vi "ScriptedStateMachine.vi"(7 "ScriptSectionName":string="Script", 8 "ErrorArray":errorcluster[](array[cluster]), 10 "script":string[](array[string]), 11 "Test.lvclass":refnum<class "Test.lvclass">) -> (0 "ErrorArray":errorcluster[](array[cluster]), 2 "Data":variant, 3 "Test.lvclass":refnum<class "Test.lvclass">)   [LabVIEW 2018, in "Test.lvclass"]
doc: "This VI sends commands to each module."
uses:
  Test.lvclass
  Test.lvclass/Test.ctl
  Typedef/BdcstInfo.ctl
  Sync/SyncPlugins/SyncPluginBase/Typedefs/clEnaTrigTmstmp.ctl
  Sync/SyncPlugins/SyncPluginBase/Typedefs/clGetTrigTmstmp.ctl
  Scope/ScopePlugins/ScopePluginBaseClass/Typedefs/Sync.ctl
  Accessors/Read ErrorSeverity.vi
  Accessors/Write ErrorSeverity.vi
  Accessors/Read ModuleIDs.vi
  Accessors/Read PluginPathArray.vi
  Accessors/Read PluginIndex.vi
  Accessors/Read LoopScript.vi
  <extravilib>/ChannelInstances/Tag-bool/Read With Abort.vi
  <extravilib>/ChannelInstances/Tag-bool/Write With Abort.vi
  <extravilib>/ChannelInstances/Tag-bool/Instantiate.vi
  <extravilib>/ChannelInstances/Tag-bool/EndpointRead.vi
  <vilib>/Utility/error.llb/Error Cluster From Error Code.vi
  <extravilib>/ChannelInstances/Tag-bool/Endpoint.vi
  <vilib>/ErrorRing/Error Ring.xnode
  <userlib>/NIST/NISTErrorLib/NISTErrorLib.lvlib
  Sync/SyncPlugins/SyncPluginBase/SyncPluginBase.lvclass
  Digitizer/DigitizerPlugins/DigitizerBaseClass/DigitizerBase.lvclass
  Sync/SyncModule/SyncModule.lvlib
  FGen/FgenModule/FgenModule.lvlib
  Digitizer/DigitizerModule/DigitizerModule.lvlib
  FGen/FgenPlugins/FgenPluginBaseClass/FgenPluginsBase.lvclass
  Analysis/AnalysisPlugins/AnalysisPluginBaseClass/AnalysisPluginsBase.lvclass
  Analysis/AnalysisModule/AnalysisModule.lvlib
  Sensor/SensorModule/SensorModule.lvlib
  Scope/ScopeModule/ScopeModule.lvlib
  Scope/ScopePlugins/ScopePluginBaseClass/ScopePluginsBase.lvclass
  AcPwr/AcPwrModule/AcPwrModule.lvlib
  <extravilib>/ChannelInstances/Tag-bool.lvlib
panel:
  out "ErrorSeverity":string
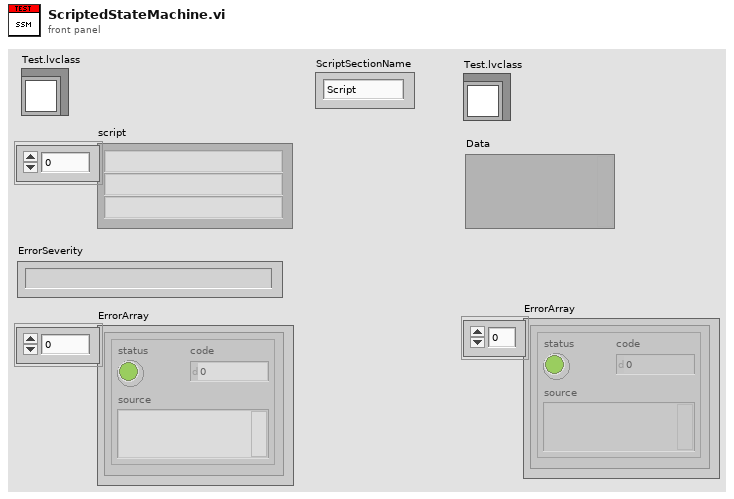
[diagram p1: front panel]
types:
  T1 = typedef "Test.lvclass/BdcstInfo.ctl" = cluster{"ModuleID":i32, "ModuleType":string, "UserEvtRef":variant, "ScriptCmd":string, "Timeout":i32}
  T2 = typedef "SyncPlugins.lvlib/SyncPluginBase.lvclass/clEnaTrigTmstmp.ctl" = cluster{"TriggerName":string, "Enable":bool}
  T3 = typedef "SyncPlugins.lvlib/SyncPluginBase.lvclass/clGetTrigTmstmp.ctl" = cluster{"TriggerName":string, "Timeout (s)":dbl}
  T4 = typedef "ScopePlugins.lvlib/ScopePluginsBase.lvclass/Sync.ctl" = cluster{"Handle":string, "SrcTerm":string, "DestTerm":string}
  T5 = typedef "Test.lvclass/FGenEventReg.ctl" = refnum<event-registration>
  T6 = typedef "Test.lvclass/ScopeEventReg.ctl" = refnum<event-registration>
  T7 = typedef "Test.lvclass/DigitizerEventReg.ctl" = refnum<event-registration>
  T8 = typedef "Test.lvclass/AcPwrEventReg.ctl" = refnum<event-registration>
  T9 = typedef "Tag-bool.lvlib/))Channel.ctl" = refnum<queue>
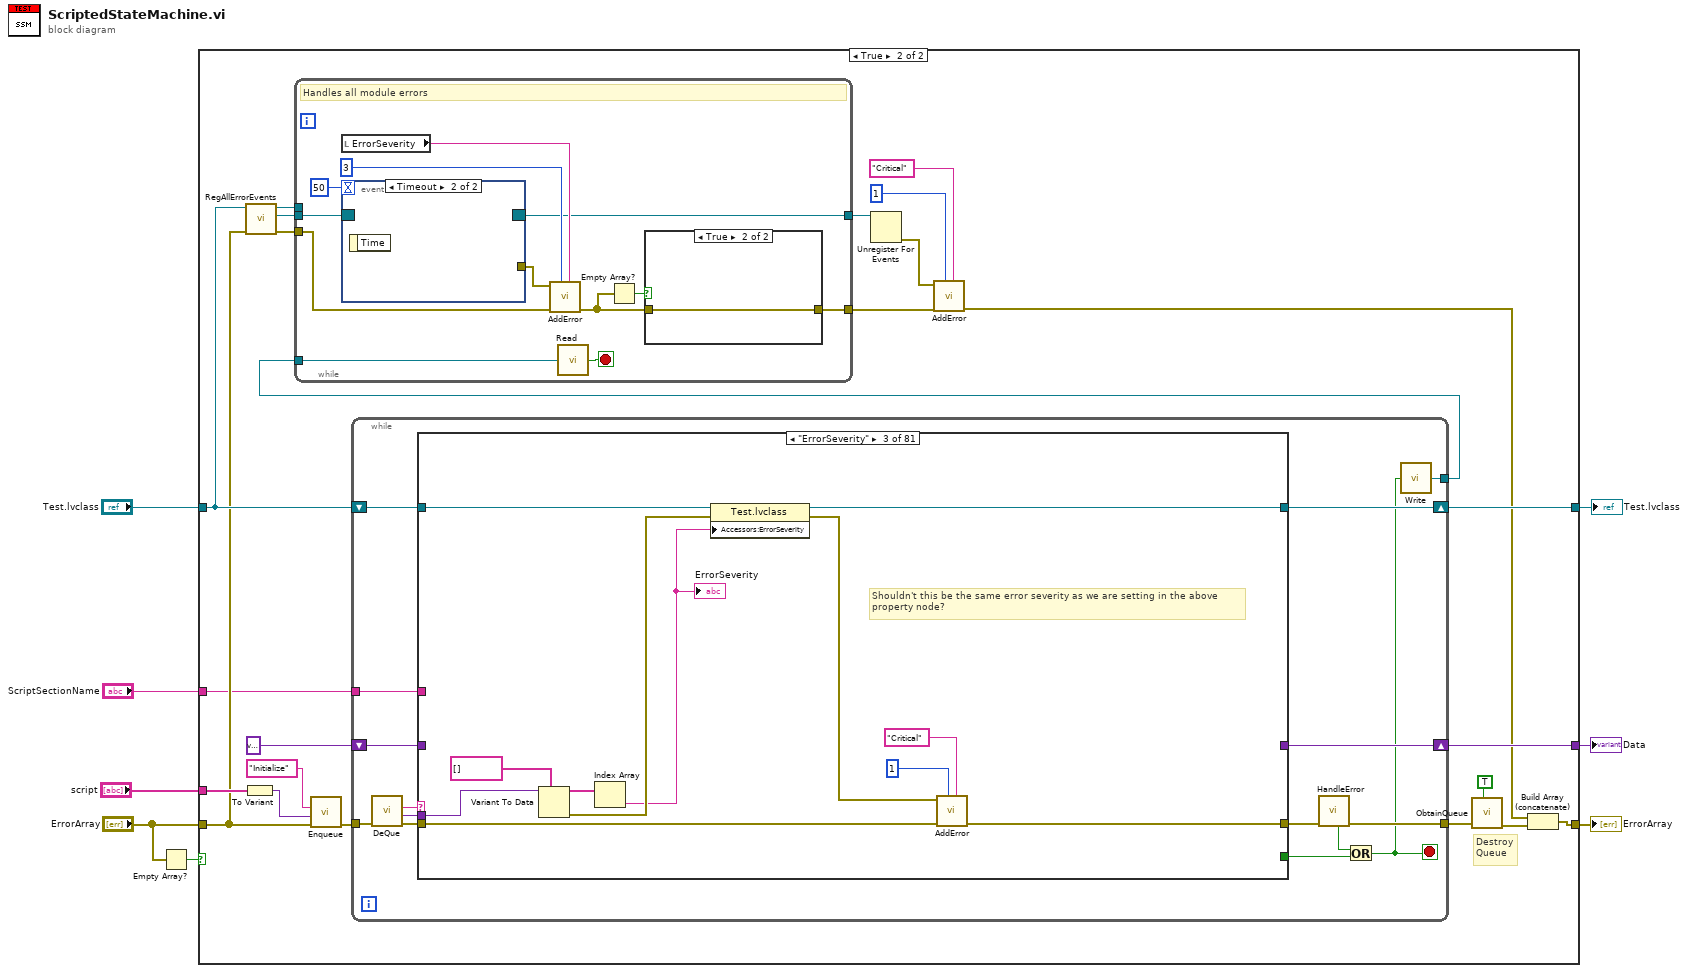
[diagram p0: block diagram]
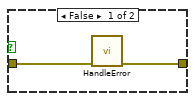
[diagram p3: hidden frame]
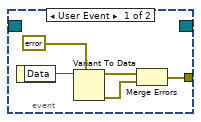
[diagram p4: hidden frame]
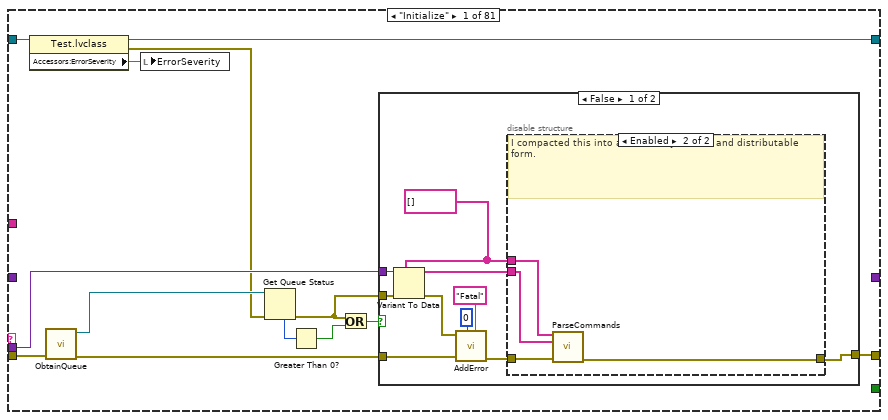
[diagram p5: hidden frame]
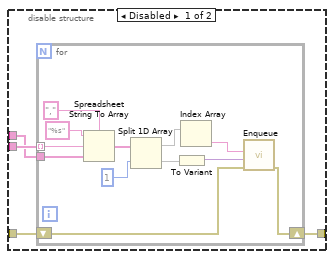
[diagram p6: hidden frame]
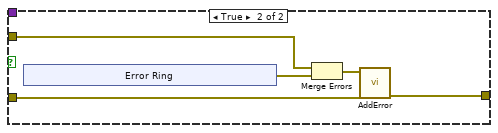
[diagram p7: hidden frame]
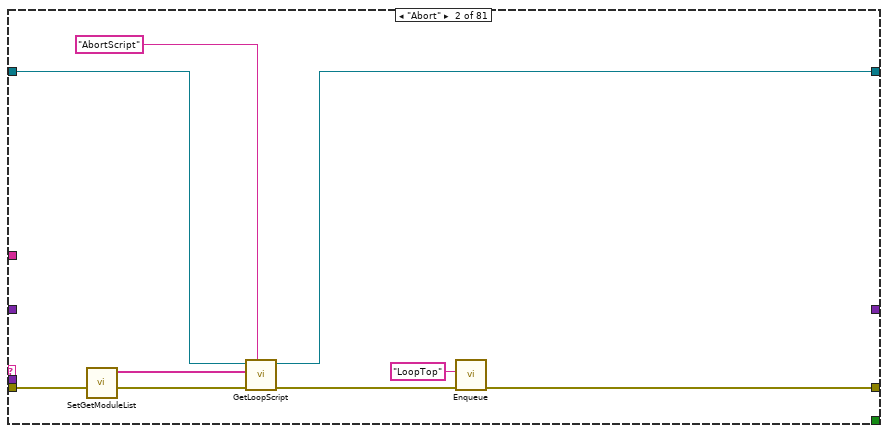
[diagram p8: hidden frame]
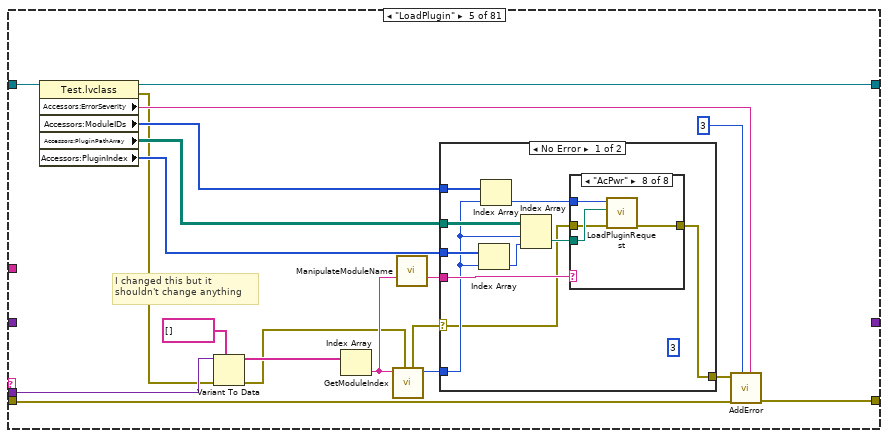
[diagram p10: hidden frame]
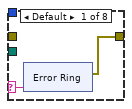
[diagram p11: hidden frame]
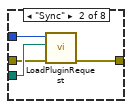
[diagram p12: hidden frame]
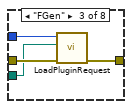
[diagram p13: hidden frame]
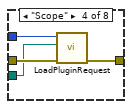
[diagram p14: hidden frame]
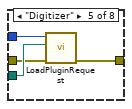
[diagram p15: hidden frame]
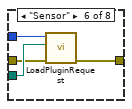
[diagram p16: hidden frame]
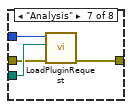
[diagram p17: hidden frame]
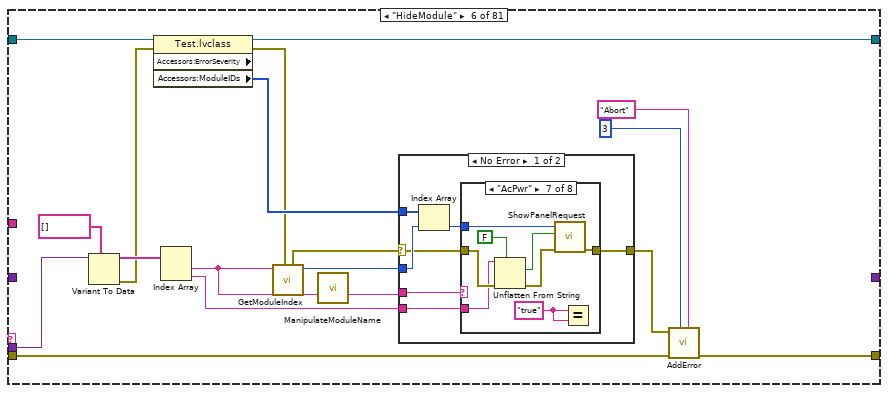
[diagram p19: hidden frame]
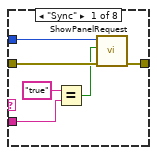
[diagram p20: hidden frame]
diagram:
  n1 = Empty Array?(array="ErrorArray") -> (empty?=w8:bool)
  n2 = case shown="True" w8 {
    tunnel: [w10 w30] -> w6
    tunnel: "Test.lvclass" -> [w10 w25]
    tunnel: "ErrorArray" -> [w9 w16]
    tunnel: [w9 w12] -> w1
    tunnel: "script" -> [_ w34]
    tunnel: [_ w29] -> w4
    tunnel: "ScriptSectionName" -> [_ w14]
    frame False {
    }
    frame True {
      # "Destroy\nQueue"
      n3 = To Variant(anything=w34) -> (Variant=w33:variant)
      n4 = call "RegAllErrorEvents.vi"("ErrorIn"=w16, "Test.lvclass"=w25) -> ("ErrorOut"=w22:errorcluster[], "Event Registration Refnum"=w23:refnum<event-registration>, "Test.lvclass"=w24:refnum<class "Test.lvclass">)  [unwired: 7 in]
      n5 = call "Enqueue.vi"("ErrorArray"=w16, "Data"=w33, "Message"="Initialize") -> ("ErrorArray"=w31:errorcluster[])  [unwired: 8 in]
      n6 = while {
        tunnel: [w68] -> w28
        tunnel: w31 -> [w67]
        shift-right: [w62] -> w30
        shift-left: w25 -> [w64]
        tunnel: w14 -> [w59]
        shift-right: [w61] -> w29
        shift-left: variant ("Data") -> [w58]
        tunnel: [w55] -> w11
        stop <- w60 stop-if-true
        n7 = call "DeQue.vi"("ErrorArray"=w67) -> ("ErrorArray"=w66:errorcluster[], "Data"=w56:variant, "Message"=w57:string)  [unwired: 8 in]
        n8 = case shown="\"ErrorSeverity\"" w57 {
          selector: w57 -> [_ _ _ _ _ _ _ _ _ _ _ _ _ _ w456 w489 _ _ w608 w651 _ _ _ _ _ _ w771 w805 _ _ _ _ _ _ _ _ w975 _ _ _ _ _ _ _ _ _ w1137 _ _ _ _ _ _ _ _ _ _ _ w1350 w1384 w1418 _ _ _ _ w1499 _ _ _ _ _ _ _ _ _ _ _ _ _ _ w1711]
          tunnel: w66 -> [w82 w130 w136 w143 w156 w218 w302 w352 w369 w385 w408 w432 w439 w447 w455 w488 w542 w563 w607 w650 w692 w708 w721 w734 w747 w760 w776 w810 w845 w859 w878 w891 w901 w914 w929 w959 w976 w1017 w1032 w1045 w1058 w1070 w1083 w1096 w1110 w1123 w1142 w1171 w1184 w1205 w1217 w1229 w1235 w1262 w1297 w1311 w1330 w1344 w1355 w1389 w1423 w1458 w1472 w1485 w1497 w1510 w1563 w1574 w1585 w1596 w1614 w1625 w1636 w1647 w1653 w1660 w1671 w1676 w1680 w1702 w1716]
          tunnel: w56 -> [w73 _ w140 _ w162 w229 w306 w354 w371 w389 w409 _ w435 w441 _ w485 w551 w564 w602 w645 w686 _ _ _ _ _ _ _ w835 w847 w873 _ _ _ w928 _ _ _ _ _ _ _ _ _ w1107 _ _ _ _ w1196 w1208 w1220 w1232 w1260 _ w1306 w1320 w1334 _ _ _ w1448 w1462 _ w1492 w1519 w1558 w1569 w1576 w1587 w1603 w1620 w1631 w1641 _ w1659 w1670 w1675 _ w1701 _]
          tunnel: [_ _ _ _ _ _ _ _ _ _ _ TRUE _ _ _ _ _ _ _ _ _ _ _ _ _ _ _ _ _ _ _ _ _ _ _ _ _ _ _ _ _ _ _ _ _ _ _ _ _ _ _ _ _ _ _ _ _ _ _ _ _ _ _ _ _ _ _ _ _ _ _ _ _ _ _ _ _ _ _ _ _] -> w65
          tunnel: w64 -> [w78 w129 w142 w144 w160 w226 w304 w353 w370 w383 w407 w433 w438 w442 w462 w490 w552 w569 w615 w657 w698 w714 w727 w740 w753 w766 w781 w815 w846 w860 w882 w894 w907 w920 w932 w962 w980 w1024 w1038 w1051 w1067 w1076 w1089 w1102 w1116 w1129 w1147 w1179 w1192 w1202 w1215 w1227 w1242 w1269 w1298 w1314 w1331 w1345 w1360 w1394 w1428 w1459 w1473 w1486 w1493 w1520 w1559 w1570 w1581 w1592 w1607 w1621 w1632 w1643 w1654 w1658 w1667 w1674 w1682 w1700 w1717]
          tunnel: [w74 w126 w133 w143 w155 w220 w301 w351 w368 w381 w398 w432 w436 w443 w454 w487 w545 w560 w606 w649 w688 w704 w717 w730 w743 w756 w770 w804 w844 w858 w875 w892 w904 w917 w930 w960 w978 w1021 w1036 w1049 w1059 w1073 w1086 w1099 w1113 w1126 w1145 w1177 w1190 w1207 w1219 w1231 w1240 w1267 w1296 w1308 w1329 w1343 w1349 w1383 w1417 w1457 w1471 w1484 w1496 w1522 w1562 w1573 w1584 w1595 w1613 w1624 w1635 w1646 w1649 w1657 w1664 w1672 w1679 w1696 w1715] -> w63
          tunnel: [w72 w128 w141 w144 w152 w224 w297 w350 w367 w376 w397 w433 w437 w442 w452 w486 w550 w559 w604 w647 w687 w703 w716 w729 w742 w755 w778 w812 w842 w856 w874 w893 w905 w918 w931 w961 w979 w1016 w1037 w1050 w1060 w1074 w1087 w1100 w1114 w1127 w1146 w1178 w1191 w1199 w1214 w1226 w1241 w1268 w1294 w1313 w1327 w1341 w1357 w1391 w1425 w1455 w1469 w1482 w1491 w1504 w1557 w1568 w1580 w1591 w1606 w1619 w1630 w1642 w1654 w1656 w1666 w1673 w1677 w1698 w1710] -> w62
          tunnel: [_ _ _ _ _ _ _ _ _ _ w392 w431 _ w440 _ _ _ _ _ _ _ _ _ _ _ _ _ _ _ _ _ _ _ _ _ _ _ _ _ _ _ _ _ _ _ _ _ _ _ w1197 w1212 w1224 w1233 _ _ _ _ _ _ _ _ _ _ _ _ _ w1545 _ _ _ _ _ _ _ _ _ _ _ _ _ _] -> w61
          tunnel: w59 -> [_ _ _ _ _ _ _ _ _ _ w393 _ _ _ _ _ _ _ _ _ _ _ _ _ _ _ _ _ _ _ _ _ _ _ _ _ _ _ _ _ _ _ _ _ _ _ _ _ _ _ _ _ _ _ _ _ _ _ _ _ _ _ _ _ _ _ _ _ _ _ _ _ _ _ _ _ _ _ _ _ _]
          tunnel: w58 -> [_ _ _ _ _ _ _ _ _ _ w392 w431 _ w440 _ _ _ _ _ _ _ _ _ _ _ _ _ _ _ _ _ _ _ _ _ _ _ _ _ _ _ _ _ _ _ _ _ _ _ _ _ _ _ _ _ _ _ _ _ _ _ _ _ _ _ _ w1545 _ _ _ _ _ _ _ _ _ _ _ _ _ _]
          frame "Initialize" {
            n9 = property class="Test.lvclass"(reference=w78) -> (reference out=w72:refnum<class "Test.lvclass">, error out=w70:errorcluster, "Accessors:ErrorSeverity"=w71:string)  [unwired: 1 in]
            n10 = call "ObtainQueue.vi"("ErrorArray"=w82) -> ("ErrorArray."=w75:errorcluster[], "TstQue"=w81:refnum<queue>)  [unwired: 9 in]
            n11 = local write "ErrorSeverity"(w71) -> ()
            n12 = Get Queue Status(queue=w81, error in (no error)=w70) -> (error out=w76:errorcluster, # elements in queue=w80:i32)  [unwired: 1 in, 6 out]
            n13 = Greater Than 0?(x=w80) -> (x > 0?=w79:bool)
            n14 = Or(x=w76, y=w79) -> (x .or. y?=w77:bool)
            n15 = case shown="False" w77 {
              tunnel: w76 -> [w92 w116]
              tunnel: w75 -> [w90 w114]
              tunnel: [w84 w113] -> w74
              tunnel: w73 -> [w91 _]
              frame False {
                w83 = string[] []
                n16 = Variant To Data(error in=w92, type=w83, Variant=w91) -> (data=w86:string[], error out=w87:errorcluster)
                n17 = call <userlib>:"AddError.vi"("Severity"="Fatal", "Priority"=u8 0, "ErrorArray"=w90, "error in (no error)"=w87) -> ("ErrorArray"=w85:errorcluster[])  [unwired: 6 in, 1 out]
                n18 = disable-structure shown="Enabled" {
                  disable-tunnel: w86 -> [w96 w109]
                  disable-tunnel: w85 -> [w95 w112]
                  disable-tunnel: w83 -> [w94 w110]
                  disable-tunnel: [w93 w111] -> w84
                  frame Disabled {
                    n19 = for {
                      tunnel: w96 -> [w106] mode=indexing
                      shift-right: [w99] -> w93
                      shift-left: w95 -> [w100]
                      tunnel: w94 -> [w105]
                      n20 = Spreadsheet String To Array(delimiter (Tab)=",", format string="%s", spreadsheet string=w106, array type (2D Dbl)=w105) -> (array=w103:string[])
                      n21 = Split 1D Array(array=w103, index=1) -> (first subarray=w98:string[], second subarray=w97:string[])
                      n22 = To Variant(anything=w97) -> (Variant=w102:variant)
                      n23 = Index Array(array=w98) -> (element=w101:string)  [unwired: 1 in]
                      n24 = call "Enqueue.vi"("ErrorArray"=w100, "Data"=w102, "Message"=w101) -> ("ErrorArray"=w99:errorcluster[])  [unwired: 8 in]
                    }
                  }
                  frame Enabled {
                    # "I compacted this into a more easy to read and distributable form."
                    n25 = call "ParseCommands.vi"("ArrayType"=w110, "SpreadSheetString"=w109, "ErrorArrayIn"=w112) -> ("ErrorArrayOut"=w111:errorcluster[])  [unwired: 10 in, 2 out]
                  }
                }
              }
              frame True {
                n26 = xnode "Error Ring"() -> ("error out"=w117:errorcluster)
                n27 = Merge Errors(w116, w117) -> (w115:errorcluster)
                n28 = call <userlib>:"AddError.vi"("ErrorArray"=w114, "error in (no error)"=w115) -> ("ErrorArray"=w113:errorcluster[])  [unwired: 8 in, 1 out]
              }
            }
          }
          frame "Abort" {
            n29 = call "SetGetModuleList.vi"() -> ("ModuleList"=w124:string[])  [unwired: 11 in]
            n30 = call "GetLoopScript.vi"("Script"="AbortScript", "ErrorArray"=w130, "ModuleNames"=w124, "Test.lvclass"=w129) -> ("ErrorArray"=w127:errorcluster[], "Test.lvclass"=w128:refnum<class "Test.lvclass">)  [unwired: 6 in]
            n31 = call "Enqueue.vi"("ErrorArray"=w127, "Message"="LoopTop") -> ("ErrorArray"=w126:errorcluster[])  [unwired: 9 in]
          }
          frame "ErrorSeverity" {
            # "Shouldn't this be the same error severity as we are setting in the above \nproperty node?"
            n32 = Variant To Data(type=string[] [], Variant=w140) -> (data=w138:string[], error out=w137:errorcluster)  [unwired: 1 in]
            n33 = Index Array(array=w138) -> (element=w131:string)  [unwired: 1 in]
            "ErrorSeverity" <- w131
            n34 = property class="Test.lvclass"(reference=w142, error in=w137, "Accessors:ErrorSeverity"=w131) -> (reference out=w141:refnum<class "Test.lvclass">, error out=w135:errorcluster)
            n35 = call <userlib>:"AddError.vi"("Severity"="Critical", "Priority"=u8 1, "ErrorArray"=w136, "error in (no error)"=w135) -> ("ErrorArray"=w133:errorcluster[])  [unwired: 6 in, 1 out]
          }
          frame "NOP" {
          }
          frame "LoadPlugin" {
            (unwired) u8 3 ("Priority")
            # "I changed this but it \nshouldn't change anything"
            n36 = property class="Test.lvclass"(reference=w160) -> (reference out=w152:refnum<class "Test.lvclass">, error out=w146:errorcluster, "Accessors:ErrorSeverity"=w154:string, "Accessors:ModuleIDs"=w159:i32[], "Accessors:PluginPathArray"=w158:path[][], "Accessors:PluginIndex"=w157:u32[])  [unwired: 1 in]
            n37 = Variant To Data(error in=w146, type=string[] [], Variant=w162) -> (data=w161:string[], error out=w147:errorcluster)
            n38 = Index Array(array=w161) -> (element=w149:string)  [unwired: 1 in]
            n39 = call "GetModuleIndex.vi"("Error In"=w147, "ModuleType"=w149) -> ("ModuleIndex"=w151:i32, "Error"=w150:errorcluster)  [unwired: 8 in]
            n40 = call "ManipulateModuleName.vi"("ModuleListSingleEntry"=w149) -> ("BeforeMatch:ModuleListSingleEntry"=w148:string)  [unwired: 9 in, 5 out]
            n41 = case shown="No Error" w150 {
              selector: w150 -> [w164 w211]
              tunnel: w159 -> [w173 _]
              tunnel: w158 -> [w172 _]
              tunnel: w157 -> [w170 _]
              tunnel: [w167 w211] -> w153
              tunnel: w148 -> [w166 _]
              tunnel: w151 -> [w165 _]
              frame No Error {
                n42 = Index Array(array=w170, index=w165) -> (element=w171:u32)
                n43 = Index Array(array=w173, index=w165) -> (element=w169:i32)
                n44 = Index Array(array=w172, index (row)=w165, index (col)=w171) -> (element=w168:path)
                n45 = case shown="\"AcPwr\"" w166 {
                  selector: w166 -> [w175 _ _ _ _ _ _ _]
                  tunnel: w169 -> [_ w186 w187 w191 w198 w202 w206 w210]
                  tunnel: w168 -> [_ w185 w188 w192 w197 w201 w205 w209]
                  tunnel: w164 -> [_ w184 w190 w194 w196 w200 w204 w208]
                  tunnel: [w174 w183 w189 w193 w195 w199 w203 w207] -> w167
                  frame Default {
                    n46 = xnode "Error Ring"("parameter 0"=w175) -> ("error out"=w174:errorcluster)
                  }
                  frame "Sync" {
                    n47 = call "LoadPluginRequest.vi"("error in (no error)"=w184, "PathToPluginINI"=w185, "ModuleID"=w186) -> ("error out"=w183:errorcluster)  [unwired: 8 in]
                  }
                  frame "FGen" {
                    n48 = call "LoadPluginRequest.vi"("error in (no error)"=w190, "PathToPluginINI"=w188, "ModuleID"=w187) -> ("error out"=w189:errorcluster)  [unwired: 8 in]
                  }
                  frame "Scope" {
                    n49 = call "LoadPluginRequest.vi"("error in (no error)"=w194, "PathToPluginINI"=w192, "ModuleID"=w191) -> ("error out"=w193:errorcluster)  [unwired: 8 in]
                  }
                  frame "Digitizer" {
                    n50 = call "LoadPluginRequest.vi"("error in (no error)"=w196, "PathToPluginINI"=w197, "ModuleID"=w198) -> ("error out"=w195:errorcluster)  [unwired: 8 in]
                  }
                  frame "Sensor" {
                    n51 = call "LoadPluginRequest.vi"("error in (no error)"=w200, "PathToPluginINI"=w201, "ModuleID"=w202) -> ("error out"=w199:errorcluster)  [unwired: 8 in]
                  }
                  frame "Analysis" {
                    n52 = call "LoadPluginRequest.vi"("error in (no error)"=w204, "PathToPluginINI"=w205, "ModuleID"=w206) -> ("error out"=w203:errorcluster)  [unwired: 8 in]
                  }
                  frame "AcPwr" {
                    n53 = call "LoadPluginRequest.vi"("error in (no error)"=w208, "PathToPluginINI"=w209, "ModuleID"=w210) -> ("error out"=w207:errorcluster)  [unwired: 8 in]
                  }
                }
              }
              frame Error {
              }
            }
            n54 = call <userlib>:"AddError.vi"("Severity"=w154, "Priority"=u8 3, "ErrorArray"=w156, "error in (no error)"=w153) -> ("ErrorArray"=w155:errorcluster[])  [unwired: 6 in, 1 out]
          }
          frame "HideModule" {
            n55 = Variant To Data(type=string[] [], Variant=w229) -> (data=w227:string[], error out=w225:errorcluster)  [unwired: 1 in]
            n56 = property class="Test.lvclass" props=["Accessors:ErrorSeverity", "Accessors:ModuleIDs"](reference=w226, error in=w225) -> (reference out=w224:refnum<class "Test.lvclass">, error out=w215:errorcluster, "Accessors:ModuleIDs"=w223:i32[])  [unwired: 1 out]
            n57 = Index Array(array=w227) -> (element #1=w212:string, element #2=w221:string)  [unwired: 2 in]
            n58 = call "GetModuleIndex.vi"("Error In"=w215, "ModuleType"=w212) -> ("ModuleIndex"=w222:i32, "Error"=w214:errorcluster)  [unwired: 8 in]
            n59 = call "ManipulateModuleName.vi"("ModuleListSingleEntry"=w212) -> ("BeforeMatch:ModuleListSingleEntry"=w213:string)  [unwired: 9 in, 5 out]
            n60 = case shown="No Error" w214 {
              selector: w214 -> [w233 w290]
              tunnel: [w230 w290] -> w219
              tunnel: w223 -> [w236 _]
              tunnel: w222 -> [w235 _]
              tunnel: w221 -> [w231 _]
              tunnel: w213 -> [w234 _]
              frame No Error {
                n61 = Index Array(array=w236, index=w235) -> (element=w232:i32)
                n62 = case shown="\"AcPwr\"" w234 {
                  selector: w234 -> [_ _ _ _ _ _ _ w281]
                  tunnel: w233 -> [w242 w248 w254 w260 w266 w272 w277 _]
                  tunnel: w232 -> [w239 w245 w251 w257 w263 w269 w280 _]
                  tunnel: [w238 w244 w250 w256 w262 w268 w279 w282] -> w230
                  tunnel: w231 -> [w237 w243 w249 w255 w261 w267 w274 _]
                  frame "Sync" {
                    n63 = Equal?(x="true", y=w237) -> (x = y?=w240:bool)
                    n64 = call "ShowPanelRequest.vi"("error in (no error)"=w242, "ShowPanel?"=w240, "ModuleID"=w239) -> ("error out"=w238:errorcluster)  [unwired: 8 in]
                  }
                  frame "FGen" {
                    n65 = Equal?(x="true", y=w243) -> (x = y?=w246:bool)
                    n66 = call "ShowPanelRequest.vi"("error in (no error)"=w248, "ShowPanel?"=w246, "ModuleID"=w245) -> ("error out"=w244:errorcluster)  [unwired: 8 in]
                  }
                  frame "Scope" {
                    n67 = Equal?(x="true", y=w249) -> (x = y?=w252:bool)
                    n68 = call "ShowPanelRequest.vi"("error in (no error)"=w254, "ShowPanel?"=w252, "ModuleID"=w251) -> ("error out"=w250:errorcluster)  [unwired: 8 in]
                  }
                  frame "Digitizer" {
                    n69 = Equal?(x="true", y=w255) -> (x = y?=w258:bool)
                    n70 = call "ShowPanelRequest.vi"("error in (no error)"=w260, "ShowPanel?"=w258, "ModuleID"=w257) -> ("error out"=w256:errorcluster)  [unwired: 8 in]
                  }
                  frame "Sensor" {
                    n71 = Equal?(x="true", y=w261) -> (x = y?=w264:bool)
                    n72 = call "ShowPanelRequest.vi"("error in (no error)"=w266, "ShowPanel?"=w264, "ModuleID"=w263) -> ("error out"=w262:errorcluster)  [unwired: 8 in]
                  }
                  frame "Analysis" {
                    n73 = Equal?(x="true", y=w267) -> (x = y?=w270:bool)
                    n74 = call "ShowPanelRequest.vi"("error in (no error)"=w272, "ShowPanel?"=w270, "ModuleID"=w269) -> ("error out"=w268:errorcluster)  [unwired: 8 in]
                  }
                  frame "AcPwr" {
                    w278 = "true" ("x")
                    n75 = Unflatten From String(type=FALSE ("ShowPanel?"), binary string=w274, error in (no error)=w277) -> (value=w273:bool, error out=w276:errorcluster)  [unwired: 2 in, 1 out]
                    n76 = call "ShowPanelRequest.vi"("error in (no error)"=w276, "ShowPanel?"=w273, "ModuleID"=w280) -> ("error out"=w279:errorcluster)  [unwired: 8 in]
                    n77 = Equal?(x=w278, y=w278) -> ()  [unwired: 1 out]
                  }
                  frame Default {
                    n78 = xnode "Error Ring"("parameter 0"=w281) -> ("error out"=w282:errorcluster)
                  }
                }
              }
              frame Error {
              }
            }
            n79 = call <userlib>:"AddError.vi"("Severity"="Abort", "Priority"=u8 3, "ErrorArray"=w218, "error in (no error)"=w219) -> ("ErrorArray"=w220:errorcluster[])  [unwired: 6 in, 1 out]
          }
          frame "PrefDlgRequest" {
            n80 = property class="Test.lvclass"(reference=w304) -> (reference out=w297:refnum<class "Test.lvclass">, error out=w291:errorcluster, "Accessors:ErrorSeverity"=w300:string, "Accessors:ModuleIDs"=w303:i32[])  [unwired: 1 in]
            n81 = Variant To Data(error in=w291, type=string[] [], Variant=w306) -> (data=w305:string[], error out=w292:errorcluster)
            n82 = Index Array(array=w305) -> (element=w294:string)  [unwired: 1 in]
            n83 = call "GetModuleIndex.vi"("Error In"=w292, "ModuleType"=w294) -> ("ModuleIndex"=w296:i32, "Error"=w295:errorcluster)  [unwired: 8 in]
            n84 = call "ManipulateModuleName.vi"("ModuleListSingleEntry"=w294) -> ("BeforeMatch:ModuleListSingleEntry"=w293:string)  [unwired: 9 in, 5 out]
            n85 = case shown="No Error" w295 {
              selector: w295 -> [w308 w344]
              tunnel: w303 -> [w313 _]
              tunnel: [w311 w344] -> w298
              tunnel: w293 -> [w310 _]
              tunnel: w296 -> [w309 _]
              frame No Error {
                n86 = Index Array(array=w313, index=w309) -> (element=w312:i32)
                n87 = case shown="\"AcPwr\"" w310 {
                  selector: w310 -> [w315 _ _ _ _ _ _ _]
                  tunnel: w312 -> [_ w325 w328 w329 w334 w337 w340 w341]
                  tunnel: w308 -> [_ w324 w327 w331 w333 w336 w339 w342]
                  tunnel: [w314 w323 w326 w330 w332 w335 w338 w343] -> w311
                  frame Default {
                    n88 = xnode "Error Ring"("parameter 0"=w315) -> ("error out"=w314:errorcluster)
                  }
                  frame "Sync" {
                    n89 = call "ConfigDlgRequest.vi"("error in (no error)"=w324, "ModuleID"=w325) -> ("error out"=w323:errorcluster)  [unwired: 9 in]
                  }
                  frame "FGen" {
                    n90 = call "ConfigDlgRequest.vi"("error in (no error)"=w327, "ModuleID"=w328) -> ("error out"=w326:errorcluster)  [unwired: 9 in]
                  }
                  frame "Scope" {
                    n91 = call "PrefDlgRequest.vi"("error in (no error)"=w331, "ModuleID"=w329) -> ("error out"=w330:errorcluster)  [unwired: 9 in]
                  }
                  frame "Digitizer" {
                    n92 = call "PrefDlgRequest.vi"("error in (no error)"=w333, "ModuleID"=w334) -> ("error out"=w332:errorcluster)  [unwired: 9 in]
                  }
                  frame "Sensor" {
                    n93 = call "ConfigureRequest.vi"("error in (no error)"=w336, "ModuleID"=w337) -> ("error out"=w335:errorcluster)  [unwired: 9 in]
                  }
                  frame "Analysis" {
                    n94 = call "ConfigDlgRequest.vi"("error in (no error)"=w339, "ModuleID"=w340) -> ("error out"=w338:errorcluster)  [unwired: 9 in]
                  }
                  frame "AcPwr" {
                    n95 = call "PrefDlgRequest.vi"("error in (no error)"=w342, "ModuleID"=w341) -> ("error out"=w343:errorcluster)  [unwired: 9 in]
                  }
                }
              }
              frame Error {
              }
            }
            n96 = call <userlib>:"AddError.vi"("Severity"=w300, "Priority"=u8 3, "ErrorArray"=w302, "error in (no error)"=w298) -> ("ErrorArray"=w301:errorcluster[])  [unwired: 6 in, 1 out]
          }
          frame "Wait" {
            n97 = property class="Test.lvclass"(reference=w353) -> (reference out=w350:refnum<class "Test.lvclass">, error out=w345:errorcluster, "Accessors:ErrorSeverity"=w349:string)  [unwired: 1 in]
            n98 = Variant To Data(type=string[] [], Variant=w354) -> (data=w356:string[], error out=w346:errorcluster)  [unwired: 1 in]
            n99 = Index Array(array=w356) -> (element=w357:string)  [unwired: 1 in]
            n100 = Decimal String To Number(string=w357) -> (number=w358:i32)  [unwired: 2 in, 1 out]
            n101 = Wait (ms)(milliseconds to wait=w358) -> ()  [unwired: 1 out]
            n102 = Merge Errors(w346, w345) -> (w347:errorcluster)
            n103 = call <userlib>:"AddError.vi"("Severity"=w349, "Priority"=u8 3, "ErrorArray"=w352, "error in (no error)"=w347) -> ("ErrorArray"=w351:errorcluster[])  [unwired: 6 in, 1 out]
          }
          frame "Delay" {
            n104 = property class="Test.lvclass"(reference=w370) -> (reference out=w367:refnum<class "Test.lvclass">, error out=w360:errorcluster, "Accessors:ErrorSeverity"=w366:string)  [unwired: 1 in]
            n105 = Variant To Data(type=string[] [], Variant=w371) -> (data=w373:string[], error out=w359:errorcluster)  [unwired: 1 in]
            n106 = Index Array(array=w373) -> (element=w364:string)  [unwired: 1 in]
            n107 = Decimal String To Number(string=w364) -> (number=w363:i32)  [unwired: 2 in, 1 out]
            n108 = To Unsigned Long Integer(number=w363) -> (unsigned 32bit integer=w362:u32)
            n109 = Wait (ms)(milliseconds to wait=w362) -> ()  [unwired: 1 out]
            n110 = Merge Errors(w359, w360) -> (w361:errorcluster)
            n111 = call <userlib>:"AddError.vi"("Severity"=w366, "Priority"=u8 3, "ErrorArray"=w369, "error in (no error)"=w361) -> ("ErrorArray"=w368:errorcluster[])  [unwired: 6 in, 1 out]
          }
          frame "Pause" {
            n112 = property class="Test.lvclass"(reference=w383) -> (reference out=w376:refnum<class "Test.lvclass">, error out=w374:errorcluster, "Accessors:ErrorSeverity"=w380:string)  [unwired: 1 in]
            n113 = Variant To Data(type=u32 0 ("milliseconds to wait"), Variant=w389) -> (data=w386:u32, error out=w382:errorcluster)  [unwired: 1 in]
            n114 = call "Enqueue.vi"("Priority? (f)"=TRUE, "ErrorArray"=w385, "Data"=w386, "Message"="Pause") -> ("ErrorArray"=w377:errorcluster[])  [unwired: 7 in]
            n115 = flat-sequence {
              tunnel: w386 -> [w391]
              tunnel: w382 -> [w390]
              tunnel: [w390] -> w378
              frame #0 {
                n116 = Wait (ms)(milliseconds to wait=w391) -> ()  [unwired: 1 out]
              }
            }
            n117 = Merge Errors(w378, w374) -> (w375:errorcluster)
            n118 = call <userlib>:"AddError.vi"("Severity"=w380, "Priority"=u8 3, "ErrorArray"=w377, "error in (no error)"=w375) -> ("ErrorArray"=w381:errorcluster[])  [unwired: 6 in, 1 out]
          }
          frame "RunTest" {
            w395 = string[] []
            # "Reverse the Script Array and Enqueue to the front of the queue.  This reverses the revesal."
            n119 = property class="Test.lvclass"(reference=w407) -> (reference out=w405:refnum<class "Test.lvclass">, error out=w394:errorcluster, "Accessors:ErrorSeverity"=w403:string)  [unwired: 1 in]
            n120 = Variant To Data(error in=w394, type=w395, Variant=w409) -> (data=w396:string[], error out=w402:errorcluster)
            n121 = call <userlib>:"AddError.vi"("Severity"=w403, "Priority"=u8 3, "ErrorArray"=w408, "error in (no error)"=w402) -> ("ErrorArray"=w404:errorcluster[])  [unwired: 6 in, 1 out]
            n122 = call "GetIniScripts.vi"("section"=w393, "ErrorArray"=w404, "ModuleNameArray"=w396, "Test.lvclass"=w405) -> ("ErrorArray"=w399:errorcluster[], "Script"=w406:string[], "Test.lvclass"=w397:refnum<class "Test.lvclass">)  [unwired: 5 in]
            n123 = Reverse 1D Array(array=w406) -> (reversed array=w400:string[])
            n124 = disable-structure shown="Enabled" {
              disable-tunnel: w400 -> [w412 w428]
              disable-tunnel: w399 -> [w411 w430]
              disable-tunnel: [w410 w429] -> w398
              disable-tunnel: w395 -> [_ w426]
              frame Disabled {
                n125 = for {
                  tunnel: w412 -> [w418] mode=indexing
                  shift-right: [w413] -> w410
                  shift-left: w411 -> [w414]
                  n126 = Spreadsheet String To Array(delimiter (Tab)=",", format string="%s", spreadsheet string=w418, array type (2D Dbl)=string[] []) -> (array=w421:string[])
                  n127 = Split 1D Array(array=w421, index=1) -> (first subarray=w422:string[], second subarray=w423:string[])
                  n128 = To Variant(anything=w423) -> (Variant=w416:variant)
                  n129 = Index Array(array=w422) -> (element=w415:string)  [unwired: 1 in]
                  n130 = call "Enqueue.vi"("Priority? (f)"=TRUE, "ErrorArray"=w414, "Data"=w416, "Message"=w415) -> ("ErrorArray"=w413:errorcluster[])  [unwired: 7 in]
                }
              }
              frame Enabled {
                n131 = call "ParseCommands.vi"("ArrayType"=w426, "Priority? (f)"=TRUE, "SpreadSheetString"=w428, "ErrorArrayIn"=w430) -> ("ErrorArrayOut"=w429:errorcluster[])  [unwired: 9 in, 2 out]
              }
            }
          }
          frame "Stop", "stop" {
          }
          frame "GetBdcst" {
            n132 = call "GetBdcst.vi"("ErrorArray"=w439, "BdcstInfo"=w435, "Test.lvclass"=w438) -> ("ErrorArray"=w436:errorcluster[], "Test.lvclass"=w437:refnum<class "Test.lvclass">)  [unwired: 7 in]
          }
          frame "GotBdcst" {
            n133 = call "DeQue.vi"("ErrorArray"=w447) -> ("ErrorArray"=w446:errorcluster[], "Message"=w445:string)  [unwired: 8 in, 1 out]
            n134 = call "Enqueue.vi"("Priority? (f)"=TRUE, "ErrorArray"=w446, "Data"=w441, "Message"=w445) -> ("ErrorArray"=w443:errorcluster[])  [unwired: 7 in]
          }
          frame "SyncGetLockStatus" {
            w457 = "Sync" ("ModuleType")
            n135 = call "GetModuleIndex.vi"("ModuleType"=w457) -> ("ModuleIndex"=w458:i32, "Error"=w461:errorcluster)  [unwired: 9 in]
            n136 = property class="Test.lvclass"(reference=w462, error in=w461) -> (reference out=w452:refnum<class "Test.lvclass">, error out=w449:errorcluster, "Accessors:ErrorSeverity"=w453:string, "Accessors:ModuleIDs"=w460:i32[])
            n137 = call "GetSyncBdcstEvents.vi"("error in (no error)"=w449) -> ("Event Registration Refnum"=w450:refnum<event-registration>, "error out"=w448:errorcluster)  [unwired: 9 in]
            n138 = Index Array(array=w460, index=w458) -> (element=w451:i32)
            n139 = call "LockToUtcIRequest.vi"("error in (no error)"=w448, "ModuleID"=w451) -> ("error out"=w459:errorcluster)  [unwired: 9 in]
            n140 = case shown="No Error" w459 {
              selector: w459 -> [_ w477]
              tunnel: w451 -> [w473 _]
              tunnel: w457 -> [w472 _]
              tunnel: w456 -> [w470 _]
              tunnel: [w466 w481] -> w454
              tunnel: w455 -> [w465 w478]
              tunnel: w453 -> [_ w480]
              tunnel: w450 -> [w463 w475]
              frame No Error {
                n141 = To Variant(anything=w463) -> (Variant=w471:variant)
                n142 = Bundle By Name(cluster=T1 {"ModuleID"=-1, "ModuleType"="", "UserEvtRef"=variant, "ScriptCmd"="", "Timeout"=5000} ("BdcstInfo"), "Timeout"=5000, "ModuleID"=w473, "ModuleType"=w472, "UserEvtRef"=w471, "ScriptCmd"=w470) -> (w468:T1)
                n143 = call "Enqueue.vi"("Priority? (f)"=TRUE, "ErrorArray"=w465, "Data"=w468, "Message"="GetBdcst") -> ("ErrorArray"=w466:errorcluster[])  [unwired: 7 in]
              }
              frame Error {
                n144 = Unregister For Events(event registration refnum=w475, error in=w477) -> (error out=w476:errorcluster)
                n145 = call <userlib>:"AddError.vi"("Severity"=w480, "Priority"=u8 3, "ErrorArray"=w478, "error in (no error)"=w476) -> ("ErrorArray"=w481:errorcluster[])  [unwired: 6 in, 1 out]
              }
            }
          }
          frame "SyncGetInfo" {
            n146 = Variant To Data(type=string[] [], Variant=w485) -> (data=w482:string[], error out=w483:errorcluster)  [unwired: 1 in]
            n147 = case shown="No Error" w483 {
              selector: w483 -> [_ w540]
              tunnel: w490 -> [w511 w539]
              tunnel: w489 -> [w505 _]
              tunnel: w488 -> [w504 w541]
              tunnel: [w503 w535] -> w487
              tunnel: [w501 w536] -> w486
              tunnel: w482 -> [w499 _]
              frame No Error {
                w506 = "Sync" ("ModuleType")
                n148 = for {
                  tunnel: w499 -> [w515] mode=indexing
                  shift-right: [w513] -> w496
                  shift-left: "" -> [w514]
                  n149 = Format Into String(format string="%s,", initial string=w514, w515) -> (resulting string=w513:string)  [unwired: 1 in, 1 out]
                }
                n150 = call "GetModuleIndex.vi"("ModuleType"=w506) -> ("ModuleIndex"=w507:i32, "Error"=w510:errorcluster)  [unwired: 9 in]
                n151 = property class="Test.lvclass"(reference=w511, error in=w510) -> (reference out=w501:refnum<class "Test.lvclass">, error out=w492:errorcluster, "Accessors:ErrorSeverity"=w502:string, "Accessors:ModuleIDs"=w509:i32[])
                n152 = String Length(string=w496) -> (length=w497:i32)
                n153 = call "GetSyncBdcstEvents.vi"("error in (no error)"=w492) -> ("Event Registration Refnum"=w493:refnum<event-registration>, "error out"=w491:errorcluster)  [unwired: 9 in]
                n154 = Index Array(array=w509, index=w507) -> (element=w500:i32)
                n155 = Decrement(x=w497) -> (x-1=w495:i32)
                n156 = String Subset(string=w496, length (rest)=w495) -> (substring=w494:string)  [unwired: 1 in]
                n157 = call "GetInfoRequest.vi"("error in (no error)"=w491, "Parameters"=w494, "ModuleID"=w500) -> ("error out"=w508:errorcluster)  [unwired: 8 in]
                n158 = case shown="No Error" w508 {
                  selector: w508 -> [_ w530]
                  tunnel: w500 -> [w526 _]
                  tunnel: w506 -> [w525 _]
                  tunnel: w505 -> [w524 _]
                  tunnel: [w520 w534] -> w503
                  tunnel: w504 -> [w519 w531]
                  tunnel: w502 -> [_ w533]
                  tunnel: w493 -> [w516 w528]
                  frame No Error {
                    n159 = To Variant(anything=w516) -> (Variant=w517:variant)
                    n160 = Bundle By Name(cluster=T1 {"ModuleID"=-1, "ModuleType"="", "UserEvtRef"=variant, "ScriptCmd"="", "Timeout"=5000} ("BdcstInfo"), "Timeout"=5000, "ModuleID"=w526, "ModuleType"=w525, "UserEvtRef"=w517, "ScriptCmd"=w524) -> (w522:T1)
                    n161 = call "Enqueue.vi"("Priority? (f)"=TRUE, "ErrorArray"=w519, "Data"=w522, "Message"="GetBdcst") -> ("ErrorArray"=w520:errorcluster[])  [unwired: 7 in]
                  }
                  frame Error {
                    n162 = Unregister For Events(event registration refnum=w528, error in=w530) -> (error out=w529:errorcluster)
                    n163 = call <userlib>:"AddError.vi"("Severity"=w533, "Priority"=u8 3, "ErrorArray"=w531, "error in (no error)"=w529) -> ("ErrorArray"=w534:errorcluster[])  [unwired: 6 in, 1 out]
                  }
                }
              }
              frame Error {
                n164 = property class="Test.lvclass"(reference=w539) -> (reference out=w536:refnum<class "Test.lvclass">, "Accessors:ErrorSeverity"=w538:string)  [unwired: 1 in, 1 out]
                n165 = call <userlib>:"AddError.vi"("Severity"=w538, "Priority"=u8 3, "ErrorArray"=w541, "error in (no error)"=w540) -> ("ErrorArray"=w535:errorcluster[])  [unwired: 6 in, 1 out]
              }
            }
          }
          frame "SyncCheckLock" {
            n166 = property class="Test.lvclass"(reference=w552) -> (reference out=w550:refnum<class "Test.lvclass">, "Accessors:ErrorSeverity"=w544:string)  [unwired: 1 in, 1 out]
            n167 = Variant To Data(type=TRUE, Variant=w551) -> (data=w546:bool, error out=w547:errorcluster)  [unwired: 1 in]
            n168 = xnode "Error Ring"() -> ("error out"=w548:errorcluster)
            n169 = Select(t=w547, s=w546, f=w548) -> (s? t:f=w543:errorcluster)
            n170 = call <userlib>:"AddError.vi"("Severity"=w544, "ErrorArray"=w542, "error in (no error)"=w543) -> ("ErrorArray"=w545:errorcluster[])  [unwired: 7 in, 1 out]
          }
          frame "SyncEnableTrigTimestamp" {
            n171 = Variant To Data(type=string[] [], Variant=w564) -> (data=w561:string[], error out=w562:errorcluster)  [unwired: 1 in]
            n172 = case shown="No Error" w562 {
              selector: w562 -> [_ w590]
              tunnel: w569 -> [w586 w589]
              tunnel: [w580 w589] -> w568
              tunnel: [w578 w590] -> w566
              tunnel: w561 -> [w577 _]
              frame No Error {
                n173 = Index Array(array=w577) -> (element #1=w575:string, element #2=w574:string)  [unwired: 2 in]
                n174 = call "GetModuleIndex.vi"("ModuleType"="Sync") -> ("ModuleIndex"=w582:i32, "Error"=w585:errorcluster)  [unwired: 9 in]
                n175 = property class="Test.lvclass"(reference=w586, error in=w585) -> (reference out=w580:refnum<class "Test.lvclass">, error out=w583:errorcluster, "Accessors:ModuleIDs"=w584:i32[])
                n176 = String Subset(string=w574, length (rest)=1 ("length (rest)")) -> (substring=w572:string)  [unwired: 1 in]
                n177 = case shown="\"True\"" w572 {
                  tunnel: [FALSE TRUE] -> w571
                  frame "False", Default {
                  }
                  frame "True" {
                  }
                }
                n178 = Bundle By Name(cluster=T2 {"TriggerName"="", "Enable"=FALSE} ("clEnaTrigTmstmp"), "TriggerName"=w575, "Enable"=w571) -> (w570:T2)
                n179 = Index Array(array=w584, index=w582) -> (element=w579:i32)
                n180 = call "EnaTrigTimestampRequest.vi"("error in (no error)"=w583, "TrigTmstmp"=w570, "ModuleID"=w579) -> ("error out"=w578:errorcluster)  [unwired: 8 in]
              }
              frame Error {
              }
            }
            n181 = property class="Test.lvclass"(reference=w568) -> (reference out=w559:refnum<class "Test.lvclass">, "Accessors:ErrorSeverity"=w558:string)  [unwired: 1 in, 1 out]
            n182 = call <userlib>:"AddError.vi"("Severity"=w558, "Priority"=u8 3, "ErrorArray"=w563, "error in (no error)"=w566) -> ("ErrorArray"=w560:errorcluster[])  [unwired: 6 in, 1 out]
          }
          frame "SyncGetTrigTimestamp" {
            w609 = "Sync" ("ModuleType")
            n183 = Variant To Data(type=string[] [], Variant=w602) -> (data=w599:string[], error out=w595:errorcluster)  [unwired: 1 in]
            n184 = call "GetModuleIndex.vi"("ModuleType"=w609) -> ("ModuleIndex"=w610:i32, "Error"=w614:errorcluster)  [unwired: 9 in]
            n185 = property class="Test.lvclass"(reference=w615, error in=w614) -> (reference out=w604:refnum<class "Test.lvclass">, error out=w612:errorcluster, "Accessors:ErrorSeverity"=w605:string, "Accessors:ModuleIDs"=w613:i32[])
            n186 = Index Array(array=w599) -> (element #1=w597:string, element #2=w598:string)  [unwired: 2 in]
            n187 = Fract/Exp String To Number(string=w598) -> (number=w594:dbl)  [unwired: 3 in, 1 out]
            n188 = Merge Errors(w612, w595) -> (w592:errorcluster)
            n189 = Index Array(array=w613, index=w610) -> (element=w603:i32)
            n190 = Bundle By Name(cluster=T3 {"TriggerName"="", "Timeout (s)"=1.0} ("TriggerName"), "TriggerName"=w597, "Timeout (s)"=w594) -> (w596:T3)
            n191 = call "GetSyncBdcstEvents.vi"("error in (no error)"=w592) -> ("Event Registration Refnum"=w593:refnum<event-registration>, "error out"=w591:errorcluster)  [unwired: 9 in]
            n192 = call "GetTrigTimestmpRequest.vi"("error in (no error)"=w591, "TriggerName"=w596, "ModuleID"=w603) -> ("error out"=w611:errorcluster)  [unwired: 8 in]
            n193 = case shown="No Error" w611 {
              selector: w611 -> [_ w631]
              tunnel: w603 -> [w627 _]
              tunnel: w609 -> [w626 _]
              tunnel: w608 -> [w624 _]
              tunnel: [w621 w635] -> w606
              tunnel: w607 -> [w620 w632]
              tunnel: w605 -> [_ w634]
              tunnel: w594 -> [w617 _]
              tunnel: w593 -> [w616 w629]
              frame No Error {
                n194 = To Variant(anything=w616) -> (Variant=w625:variant)
                n195 = To Long Integer(number=w617) -> (32bit integer=w618:i32)
                n196 = Bundle By Name(cluster=T1 {"ModuleID"=-1, "ModuleType"="", "UserEvtRef"=variant, "ScriptCmd"="", "Timeout"=5000} ("BdcstInfo"), "Timeout"=w618, "ModuleID"=w627, "ModuleType"=w626, "UserEvtRef"=w625, "ScriptCmd"=w624) -> (w623:T1)
                n197 = call "Enqueue.vi"("Priority? (f)"=TRUE, "ErrorArray"=w620, "Data"=w623, "Message"="GetBdcst") -> ("ErrorArray"=w621:errorcluster[])  [unwired: 7 in]
              }
              frame Error {
                n198 = Unregister For Events(event registration refnum=w629, error in=w631) -> (error out=w630:errorcluster)
                n199 = call <userlib>:"AddError.vi"("Severity"=w634, "Priority"=u8 3, "ErrorArray"=w632, "error in (no error)"=w630) -> ("ErrorArray"=w635:errorcluster[])  [unwired: 6 in, 1 out]
              }
            }
          }
          frame "SyncGetPpsTime" {
            w652 = "Sync" ("ModuleType")
            n200 = Variant To Data(type=string[] [], Variant=w645) -> (data=w643:string[], error out=w639:errorcluster)  [unwired: 1 in]
            n201 = call "GetModuleIndex.vi"("ModuleType"=w652) -> ("ModuleIndex"=w653:i32, "Error"=w656:errorcluster)  [unwired: 9 in]
            n202 = property class="Test.lvclass"(reference=w657, error in=w656) -> (reference out=w647:refnum<class "Test.lvclass">, error out=w641:errorcluster, "Accessors:ErrorSeverity"=w648:string, "Accessors:ModuleIDs"=w655:i32[])
            n203 = Index Array(array=w643) -> (element=w640:string)  [unwired: 1 in]
            n204 = Fract/Exp String To Number(string=w640) -> (number=w642:dbl)  [unwired: 3 in, 1 out]
            n205 = Index Array(array=w655, index=w653) -> (element=w646:i32)
            n206 = Merge Errors(w641, w639) -> (w637:errorcluster)
            n207 = call "GetSyncBdcstEvents.vi"("error in (no error)"=w637) -> ("Event Registration Refnum"=w638:refnum<event-registration>, "error out"=w636:errorcluster)  [unwired: 9 in]
            n208 = call "TriggerTimeRequest.vi"("error in (no error)"=w636, "ModuleID"=w646) -> ("error out"=w654:errorcluster)  [unwired: 9 in]
            n209 = case shown="Error" w654 {
              selector: w654 -> [_ w673]
              tunnel: w646 -> [w669 _]
              tunnel: w652 -> [w668 _]
              tunnel: w651 -> [w666 _]
              tunnel: [w663 w677] -> w649
              tunnel: w650 -> [w662 w674]
              tunnel: w648 -> [_ w676]
              tunnel: w642 -> [w659 _]
              tunnel: w638 -> [w658 w671]
              frame No Error {
                n210 = To Variant(anything=w658) -> (Variant=w667:variant)
                n211 = To Long Integer(number=w659) -> (32bit integer=w660:i32)
                n212 = Bundle By Name(cluster=T1 {"ModuleID"=-1, "ModuleType"="", "UserEvtRef"=variant, "ScriptCmd"="", "Timeout"=5000} ("BdcstInfo"), "Timeout"=w660, "ModuleID"=w669, "ModuleType"=w668, "UserEvtRef"=w667, "ScriptCmd"=w666) -> (w665:T1)
                n213 = call "Enqueue.vi"("Priority? (f)"=TRUE, "ErrorArray"=w662, "Data"=w665, "Message"="GetBdcst") -> ("ErrorArray"=w663:errorcluster[])  [unwired: 7 in]
              }
              frame Error {
                n214 = Unregister For Events(event registration refnum=w671, error in=w673) -> (error out=w672:errorcluster)
                n215 = call <userlib>:"AddError.vi"("Severity"=w676, "Priority"=u8 3, "ErrorArray"=w674, "error in (no error)"=w672) -> ("ErrorArray"=w677:errorcluster[])  [unwired: 6 in, 1 out]
              }
            }
          }
          frame "FGenInitialize" {
            n216 = Variant To Data(type=string[] [], Variant=w686) -> (data=w683:string[])  [unwired: 1 in, 1 out]
            n217 = for {
              tunnel: w683 -> [w701] mode=indexing
              tunnel: [w699] -> w682 mode=indexing
              n218 = Equal?(x=w701, y="true") -> (x = y?=w699:bool)
            }
            n219 = Index Array(array=w683, index #1=0 ("index")) -> ()  [unwired: 1 in, 2 out]
            n220 = call "GetModuleIndex.vi"("ModuleType"="FGen") -> ("ModuleIndex"=w695:i32, "Error"=w679:errorcluster)  [unwired: 9 in]
            n221 = property class="Test.lvclass"(reference=w698, error in=w679) -> (reference out=w687:refnum<class "Test.lvclass">, error out=w693:errorcluster, "Accessors:ErrorSeverity"=w690:string, "Accessors:ModuleIDs"=w696:i32[])
            n222 = Index Array(array=w682, index #1=0 ("index")) -> (element #1=w680:bool, element #2=w678:bool)  [unwired: 1 in]
            n223 = Index Array(array=w696, index=w695) -> (element=w694:i32)
            n224 = call "InitializeRequest.vi"("error in (no error)"=w693, "Reset"=w678, "IDQuery"=w680, "ModuleID"=w694) -> ("error out"=w691:errorcluster)  [unwired: 7 in]
            n225 = call <userlib>:"AddError.vi"("Severity"=w690, "Priority"=u8 3, "ErrorArray"=w692, "error in (no error)"=w691) -> ("ErrorArray"=w688:errorcluster[])  [unwired: 6 in, 1 out]
          }
          frame "FGenConfigFunction" {
            n226 = call "GetModuleIndex.vi"("ModuleType"="FGen") -> ("ModuleIndex"=w711:i32, "Error"=w702:errorcluster)  [unwired: 9 in]
            n227 = property class="Test.lvclass"(reference=w714, error in=w702) -> (reference out=w703:refnum<class "Test.lvclass">, error out=w709:errorcluster, "Accessors:ErrorSeverity"=w706:string, "Accessors:ModuleIDs"=w712:i32[])
            n228 = Index Array(array=w712, index=w711) -> (element=w710:i32)
            n229 = call "ConfigFunctionRequest.vi"("error in (no error)"=w709, "ModuleID"=w710) -> ("error out"=w707:errorcluster)  [unwired: 9 in]
            n230 = call <userlib>:"AddError.vi"("Severity"=w706, "Priority"=u8 3, "ErrorArray"=w708, "error in (no error)"=w707) -> ("ErrorArray"=w704:errorcluster[])  [unwired: 6 in, 1 out]
          }
          frame "FGenConfigTriggers" {
            n231 = call "GetModuleIndex.vi"("ModuleType"="FGen") -> ("ModuleIndex"=w724:i32, "Error"=w715:errorcluster)  [unwired: 9 in]
            n232 = property class="Test.lvclass"(reference=w727, error in=w715) -> (reference out=w716:refnum<class "Test.lvclass">, error out=w722:errorcluster, "Accessors:ErrorSeverity"=w719:string, "Accessors:ModuleIDs"=w725:i32[])
            n233 = Index Array(array=w725, index=w724) -> (element=w723:i32)
            n234 = call "ConfigTriggersRequest.vi"("error in (no error)"=w722, "ModuleID"=w723) -> ("error out"=w720:errorcluster)  [unwired: 9 in]
            n235 = call <userlib>:"AddError.vi"("Severity"=w719, "Priority"=u8 3, "ErrorArray"=w721, "error in (no error)"=w720) -> ("ErrorArray"=w717:errorcluster[])  [unwired: 6 in, 1 out]
          }
          frame "FGenInitiateGen" {
            n236 = call "GetModuleIndex.vi"("ModuleType"="FGen") -> ("ModuleIndex"=w737:i32, "Error"=w728:errorcluster)  [unwired: 9 in]
            n237 = property class="Test.lvclass"(reference=w740, error in=w728) -> (reference out=w729:refnum<class "Test.lvclass">, error out=w735:errorcluster, "Accessors:ErrorSeverity"=w732:string, "Accessors:ModuleIDs"=w738:i32[])
            n238 = Index Array(array=w738, index=w737) -> (element=w736:i32)
            n239 = call "InitGenRequest.vi"("error in (no error)"=w735, "ModuleID"=w736) -> ("error out"=w733:errorcluster)  [unwired: 9 in]
            n240 = call <userlib>:"AddError.vi"("Severity"=w732, "Priority"=u8 3, "ErrorArray"=w734, "error in (no error)"=w733) -> ("ErrorArray"=w730:errorcluster[])  [unwired: 6 in, 1 out]
          }
          frame "FGenAbortGen" {
            n241 = call "GetModuleIndex.vi"("ModuleType"="FGen") -> ("ModuleIndex"=w750:i32, "Error"=w741:errorcluster)  [unwired: 9 in]
            n242 = property class="Test.lvclass"(reference=w753, error in=w741) -> (reference out=w742:refnum<class "Test.lvclass">, error out=w748:errorcluster, "Accessors:ErrorSeverity"=w745:string, "Accessors:ModuleIDs"=w751:i32[])
            n243 = Index Array(array=w751, index=w750) -> (element=w749:i32)
            n244 = call "AbortGenRequest.vi"("error in (no error)"=w748, "ModuleID"=w749) -> ("error out"=w746:errorcluster)  [unwired: 9 in]
            n245 = call <userlib>:"AddError.vi"("Severity"=w745, "Priority"=u8 3, "ErrorArray"=w747, "error in (no error)"=w746) -> ("ErrorArray"=w743:errorcluster[])  [unwired: 6 in, 1 out]
          }
          frame "FGenClose" {
            n246 = call "GetModuleIndex.vi"("ModuleType"="FGen") -> ("ModuleIndex"=w763:i32, "Error"=w754:errorcluster)  [unwired: 9 in]
            n247 = property class="Test.lvclass"(reference=w766, error in=w754) -> (reference out=w755:refnum<class "Test.lvclass">, error out=w761:errorcluster, "Accessors:ErrorSeverity"=w758:string, "Accessors:ModuleIDs"=w764:i32[])
            n248 = Index Array(array=w764, index=w763) -> (element=w762:i32)
            n249 = call "CloseRequest.vi"("error in (no error)"=w761, "ModuleID"=w762) -> ("error out"=w759:errorcluster)  [unwired: 9 in]
            n250 = call <userlib>:"AddError.vi"("Severity"=w758, "Priority"=u8 3, "ErrorArray"=w760, "error in (no error)"=w759) -> ("ErrorArray"=w756:errorcluster[])  [unwired: 6 in, 1 out]
          }
          frame "FGenGetFunctionClass" {
            w772 = "FGen"
            n251 = call "GetModuleIndex.vi"("ModuleType"=w772) -> ("ModuleIndex"=w779:i32, "Error"=w777:errorcluster)  [unwired: 9 in]
            n252 = property class="Test.lvclass"(reference=w781, error in=w777) -> (reference out=w778:refnum<class "Test.lvclass">, error out=w768:errorcluster, "Accessors:ErrorSeverity"=w774:string, "Accessors:ModuleIDs"=w780:i32[])
            n253 = Index Array(array=w780, index=w779) -> (element=w773:i32)
            n254 = call "GetFGenBdcstEvents.vi"("error in (no error)"=w768) -> ("Event Registration Refnum"=w769:T5, "error out"=w767:errorcluster)  [unwired: 9 in]
            n255 = call "GetFunctionRequest.vi"("error in (no error)"=w767, "ModuleID"=w773) -> ("error out"=w775:errorcluster)  [unwired: 9 in]
            n256 = case shown="No Error" w775 {
              selector: w775 -> [_ w796]
              tunnel: w773 -> [w792 _]
              tunnel: w772 -> [w791 _]
              tunnel: w771 -> [w789 _]
              tunnel: [w785 w800] -> w770
              tunnel: w776 -> [w784 w797]
              tunnel: w774 -> [_ w799]
              tunnel: w769 -> [w782 w794]
              frame No Error {
                n257 = To Variant(anything=w782) -> (Variant=w790:variant)
                n258 = Bundle By Name(cluster=T1 {"ModuleID"=-1, "ModuleType"="", "UserEvtRef"=variant, "ScriptCmd"="", "Timeout"=5000} ("BdcstInfo"), "Timeout"=5000, "ModuleID"=w792, "ModuleType"=w791, "UserEvtRef"=w790, "ScriptCmd"=w789) -> (w787:T1)
                n259 = call "Enqueue.vi"("Priority? (f)"=TRUE, "ErrorArray"=w784, "Data"=w787, "Message"="GetBdcst") -> ("ErrorArray"=w785:errorcluster[])  [unwired: 7 in]
              }
              frame Error {
                n260 = Unregister For Events(event registration refnum=w794, error in=w796) -> (error out=w795:errorcluster)
                n261 = call <userlib>:"AddError.vi"("Severity"=w799, "Priority"=u8 3, "ErrorArray"=w797, "error in (no error)"=w795) -> ("ErrorArray"=w800:errorcluster[])  [unwired: 6 in, 1 out]
              }
            }
          }
          frame "FGenGetFunctionParams" {
            w806 = "FGen"
            n262 = call "GetModuleIndex.vi"("ModuleType"=w806) -> ("ModuleIndex"=w813:i32, "Error"=w811:errorcluster)  [unwired: 9 in]
            n263 = property class="Test.lvclass"(reference=w815, error in=w811) -> (reference out=w812:refnum<class "Test.lvclass">, error out=w802:errorcluster, "Accessors:ErrorSeverity"=w808:string, "Accessors:ModuleIDs"=w814:i32[])
            n264 = Index Array(array=w814, index=w813) -> (element=w807:i32)
            n265 = call "GetFGenBdcstEvents.vi"("error in (no error)"=w802) -> ("Event Registration Refnum"=w803:T5, "error out"=w801:errorcluster)  [unwired: 9 in]
            n266 = call "GetFunctionParamsRequest.vi"("error in (no error)"=w801, "ModuleID"=w807) -> ("error out"=w809:errorcluster)  [unwired: 9 in]
            n267 = case shown="No Error" w809 {
              selector: w809 -> [_ w831]
              tunnel: w807 -> [w826 _]
              tunnel: w806 -> [w825 _]
              tunnel: w805 -> [w823 _]
              tunnel: [w819 w832] -> w804
              tunnel: w810 -> [w818 w828]
              tunnel: w808 -> [_ w830]
              tunnel: w803 -> [w816 _]
              frame No Error {
                n268 = To Variant(anything=w816) -> (Variant=w824:variant)
                n269 = Bundle By Name(cluster=T1 {"ModuleID"=-1, "ModuleType"="", "UserEvtRef"=variant, "ScriptCmd"="", "Timeout"=5000} ("BdcstInfo"), "Timeout"=10000, "ModuleID"=w826, "ModuleType"=w825, "UserEvtRef"=w824, "ScriptCmd"=w823) -> (w821:T1)
                n270 = call "Enqueue.vi"("Priority? (f)"=TRUE, "ErrorArray"=w818, "Data"=w821, "Message"="GetBdcst") -> ("ErrorArray"=w819:errorcluster[])  [unwired: 7 in]
              }
              frame Error {
                n271 = call <userlib>:"AddError.vi"("Severity"=w830, "Priority"=u8 3, "ErrorArray"=w828, "error in (no error)"=w831) -> ("ErrorArray"=w832:errorcluster[])  [unwired: 6 in, 1 out]
              }
            }
          }
          frame "FGenSetFunctionClass" {
            n272 = call "GetModuleIndex.vi"("ModuleType"="FGen") -> ("ModuleIndex"=w839:i32, "Error"=w834:errorcluster)  [unwired: 9 in]
            n273 = property class="Test.lvclass"(reference=w846, error in=w834) -> (reference out=w842:refnum<class "Test.lvclass">, error out=w833:errorcluster, "Accessors:ErrorSeverity"=w837:string, "Accessors:ModuleIDs"=w840:i32[])
            n274 = Index Array(array=w840, index=w839) -> (element=w838:i32)
            n275 = call "SetFunctionRequest.vi"("error in (no error)"=w833, "FunctionConfig"=w835, "ModuleID"=w838) -> ("error out"=w843:errorcluster)  [unwired: 8 in]
            n276 = call <userlib>:"AddError.vi"("Severity"=w837, "Priority"=u8 3, "ErrorArray"=w845, "error in (no error)"=w843) -> ("ErrorArray"=w844:errorcluster[])  [unwired: 6 in, 1 out]
          }
          frame "FGenSetFunctionParams" {
            n277 = call "GetModuleIndex.vi"("ModuleType"="FGen") -> ("ModuleIndex"=w853:i32, "Error"=w849:errorcluster)  [unwired: 9 in]
            n278 = property class="Test.lvclass"(reference=w860, error in=w849) -> (reference out=w856:refnum<class "Test.lvclass">, error out=w848:errorcluster, "Accessors:ErrorSeverity"=w851:string, "Accessors:ModuleIDs"=w854:i32[])
            n279 = Index Array(array=w854, index=w853) -> (element=w852:i32)
            n280 = call "SetFunctionParamsRequest.vi"("error in (no error)"=w848, "FunctionConfig"=w847, "ModuleID"=w852) -> ("error out"=w857:errorcluster)  [unwired: 8 in]
            n281 = call <userlib>:"AddError.vi"("Severity"=w851, "Priority"=u8 3, "ErrorArray"=w859, "error in (no error)"=w857) -> ("ErrorArray"=w858:errorcluster[])  [unwired: 6 in, 1 out]
          }
          frame "ScopeInitialize" {
            n282 = Variant To Data(type=string[] [], Variant=w873) -> (data=w870:string[])  [unwired: 1 in, 1 out]
            n283 = for {
              tunnel: w870 -> [w885] mode=indexing
              tunnel: [w883] -> w869 mode=indexing
              n284 = Equal?(x=w885, y="true") -> (x = y?=w883:bool)
            }
            n285 = Index Array(array=w870, index #1=0 ("index")) -> ()  [unwired: 1 in, 2 out]
            n286 = call "GetModuleIndex.vi"("ModuleType"="Scope") -> ("ModuleIndex"=w879:i32, "Error"=w867:errorcluster)  [unwired: 9 in]
            n287 = property class="Test.lvclass"(reference=w882, error in=w867) -> (reference out=w874:refnum<class "Test.lvclass">, error out=w865:errorcluster, "Accessors:ErrorSeverity"=w877:string, "Accessors:ModuleIDs"=w880:i32[])
            n288 = Index Array(array=w869, index #1=0 ("index")) -> (element #1=w863:bool, element #2=w862:bool)  [unwired: 1 in]
            n289 = Bundle(w862, w863) -> (w861:cluster{bool, bool})  [unwired: 1 in]
            n290 = Index Array(array=w880, index=w879) -> (element=w866:i32)
            n291 = call "InitializeRequest.vi"("error in (no error)"=w865, "InitOptions"=w861, "ModuleID"=w866) -> ("error out"=w864:errorcluster)  [unwired: 8 in]
            n292 = call <userlib>:"AddError.vi"("Severity"=w877, "Priority"=u8 3, "ErrorArray"=w878, "error in (no error)"=w864) -> ("ErrorArray"=w875:errorcluster[])  [unwired: 6 in, 1 out]
          }
          frame "ScopeConfigAcquisition" {
            n293 = call "GetModuleIndex.vi"("ModuleType"="Scope") -> ("ModuleIndex"=w895:i32, "Error"=w897:errorcluster)  [unwired: 9 in]
            n294 = property class="Test.lvclass"(reference=w894, error in=w897) -> (reference out=w893:refnum<class "Test.lvclass">, error out=w886:errorcluster, "Accessors:ErrorSeverity"=w890:string, "Accessors:ModuleIDs"=w896:i32[])
            n295 = Index Array(array=w896, index=w895) -> (element=w888:i32)
            n296 = call "ConfigAquisitionRequest.vi"("error in (no error)"=w886, "ModuleID"=w888) -> ("error out"=w887:errorcluster)  [unwired: 9 in]
            n297 = call <userlib>:"AddError.vi"("Severity"=w890, "Priority"=u8 3, "ErrorArray"=w891, "error in (no error)"=w887) -> ("ErrorArray"=w892:errorcluster[])  [unwired: 6 in, 1 out]
          }
          frame "ScopeConfigChannels" {
            n298 = call "GetModuleIndex.vi"("ModuleType"="Scope") -> ("ModuleIndex"=w908:i32, "Error"=w910:errorcluster)  [unwired: 9 in]
            n299 = property class="Test.lvclass"(reference=w907, error in=w910) -> (reference out=w905:refnum<class "Test.lvclass">, error out=w902:errorcluster, "Accessors:ErrorSeverity"=w900:string, "Accessors:ModuleIDs"=w909:i32[])
            n300 = Index Array(array=w909, index=w908) -> (element=w906:i32)
            n301 = call "ConfigChannelsRequest.vi"("error in (no error)"=w902, "ModuleID"=w906) -> ("error out"=w903:errorcluster)  [unwired: 9 in]
            n302 = call <userlib>:"AddError.vi"("Severity"=w900, "Priority"=u8 3, "ErrorArray"=w901, "error in (no error)"=w903) -> ("ErrorArray"=w904:errorcluster[])  [unwired: 6 in, 1 out]
          }
          frame "ScopeConfigTrigger" {
            n303 = call "GetModuleIndex.vi"("ModuleType"="Scope") -> ("ModuleIndex"=w921:i32, "Error"=w923:errorcluster)  [unwired: 9 in]
            n304 = property class="Test.lvclass"(reference=w920, error in=w923) -> (reference out=w918:refnum<class "Test.lvclass">, error out=w915:errorcluster, "Accessors:ErrorSeverity"=w913:string, "Accessors:ModuleIDs"=w922:i32[])
            n305 = Index Array(array=w922, index=w921) -> (element=w919:i32)
            n306 = call "ConfigTriggerRequest.vi"("error in (no error)"=w915, "ModuleID"=w919) -> ("error out"=w916:errorcluster)  [unwired: 9 in]
            n307 = call <userlib>:"AddError.vi"("Severity"=w913, "Priority"=u8 3, "ErrorArray"=w914, "error in (no error)"=w916) -> ("ErrorArray"=w917:errorcluster[])  [unwired: 6 in, 1 out]
          }
          frame "ScopeSetSync" {
            n308 = Variant To Data(type=string[] [], Variant=w928) -> (data=w926:string[], error out=w925:errorcluster)  [unwired: 1 in]
            n309 = case shown="No Error" w925 {
              tunnel: w932 -> [w947 w952]
              tunnel: [w946 w952] -> w931
              tunnel: [w945 w953] -> w930
              tunnel: w929 -> [w942 w953]
              tunnel: w926 -> [w939 _]
              frame No Error {
                n310 = Index Array(array=w939) -> (element #1=w937:string, element #2=w936:string, element #3=w935:string)  [unwired: 3 in]
                n311 = Bundle By Name(cluster=T4 {"Handle"="", "SrcTerm"="", "DestTerm"=""} ("Sync"), "Handle"=w937, "SrcTerm"=w936, "DestTerm"=w935) -> (w933:T4)
                n312 = call "GetModuleIndex.vi"("ModuleType"="Scope") -> ("ModuleIndex"=w948:i32, "Error"=w950:errorcluster)  [unwired: 9 in]
                n313 = property class="Test.lvclass"(reference=w947, error in=w950) -> (reference out=w946:refnum<class "Test.lvclass">, error out=w943:errorcluster, "Accessors:ErrorSeverity"=w941:string, "Accessors:ModuleIDs"=w949:i32[])
                n314 = Index Array(array=w949, index=w948) -> (element=w934:i32)
                n315 = call "SetSyncRequest.vi"("error in (no error)"=w943, "Sync"=w933, "ModuleID"=w934) -> ("error out"=w944:errorcluster)  [unwired: 8 in]
                n316 = call <userlib>:"AddError.vi"("Severity"=w941, "Priority"=u8 3, "ErrorArray"=w942, "error in (no error)"=w944) -> ("ErrorArray"=w945:errorcluster[])  [unwired: 6 in, 1 out]
              }
              frame Error {
              }
            }
          }
          frame "ScopeFetchWaveforms" {
            n317 = call "GetModuleIndex.vi"("ModuleType"="Scope") -> ("ModuleIndex"=w963:i32, "Error"=w965:errorcluster)  [unwired: 9 in]
            n318 = property class="Test.lvclass"(reference=w962, error in=w965) -> (reference out=w961:refnum<class "Test.lvclass">, error out=w955:errorcluster, "Accessors:ErrorSeverity"=w958:string, "Accessors:ModuleIDs"=w964:i32[])
            n319 = Index Array(array=w964, index=w963) -> (element=w956:i32)
            n320 = call "FetchWaveformRequest.vi"("error in (no error)"=w955, "ModuleID"=w956) -> ("error out"=w954:errorcluster)  [unwired: 9 in]
            n321 = call <userlib>:"AddError.vi"("Severity"=w958, "Priority"=u8 3, "ErrorArray"=w959, "error in (no error)"=w954) -> ("ErrorArray"=w960:errorcluster[])  [unwired: 6 in, 1 out]
          }
          frame "ScopeReadWaveforms" {
            w972 = "Scope" ("ModuleType")
            n322 = call "GetModuleIndex.vi"("ModuleType"=w972) -> ("ModuleIndex"=w981:i32, "Error"=w983:errorcluster)  [unwired: 9 in]
            n323 = property class="Test.lvclass"(reference=w980, error in=w983) -> (reference out=w979:refnum<class "Test.lvclass">, error out=w968:errorcluster, "Accessors:ErrorSeverity"=w973:string, "Accessors:ModuleIDs"=w982:i32[])
            n324 = Index Array(array=w982, index=w981) -> (element=w971:i32)
            n325 = call "GetScopeBrdcstEvents.vi"("error in (no error)"=w968) -> ("Event Registration Refnum"=w969:T6, "error out"=w967:errorcluster)  [unwired: 9 in]
            n326 = call "ReadWaveformRequest.vi"("error in (no error)"=w967, "ModuleID"=w971) -> ("error out"=w970:errorcluster)  [unwired: 9 in]
            n327 = disable-structure shown="Enabled" {
              disable-tunnel: w976 -> [w991 w1014]
              disable-tunnel: w975 -> [w990 _]
              disable-tunnel: [w989 w1015] -> w974
              disable-tunnel: w973 -> [w988 w1012]
              disable-tunnel: w972 -> [w987 _]
              disable-tunnel: w971 -> [w986 _]
              disable-tunnel: w970 -> [w985 w1013]
              disable-tunnel: w969 -> [w984 _]
              frame Enabled {
                n328 = case shown="No Error" w985 {
                  selector: w985 -> [_ w1006]
                  tunnel: w986 -> [w1002 _]
                  tunnel: w987 -> [w1001 _]
                  tunnel: w990 -> [w1000 _]
                  tunnel: [w996 w1010] -> w989
                  tunnel: w991 -> [w995 w1007]
                  tunnel: w988 -> [_ w1009]
                  tunnel: w984 -> [w992 w1004]
                  frame No Error {
                    n329 = To Variant(anything=w992) -> (Variant=w993:variant)
                    n330 = Bundle By Name(cluster=T1 {"ModuleID"=-1, "ModuleType"="", "UserEvtRef"=variant, "ScriptCmd"="", "Timeout"=5000} ("BdcstInfo"), "Timeout"=5000, "ModuleID"=w1002, "ModuleType"=w1001, "UserEvtRef"=w993, "ScriptCmd"=w1000) -> (w998:T1)
                    n331 = call "Enqueue.vi"("Priority? (f)"=TRUE, "ErrorArray"=w995, "Data"=w998, "Message"="GetBdcst") -> ("ErrorArray"=w996:errorcluster[])  [unwired: 7 in]
                  }
                  frame Error {
                    n332 = Unregister For Events(event registration refnum=w1004, error in=w1006) -> (error out=w1005:errorcluster)
                    n333 = call <userlib>:"AddError.vi"("Severity"=w1009, "Priority"=u8 3, "ErrorArray"=w1007, "error in (no error)"=w1005) -> ("ErrorArray"=w1010:errorcluster[])  [unwired: 6 in, 1 out]
                  }
                }
              }
              frame Disabled {
                n334 = call <userlib>:"AddError.vi"("Severity"=w1012, "Priority"=u8 3, "ErrorArray"=w1014, "error in (no error)"=w1013) -> ("ErrorArray"=w1015:errorcluster[])  [unwired: 6 in, 1 out]
              }
            }
            n335 = call <userlib>:"AddError.vi"("Severity"=w973, "Priority"=u8 3, "ErrorArray"=w974) -> ("ErrorArray"=w978:errorcluster[])  [unwired: 7 in, 1 out]
          }
          frame "ScopeStopAcquisition" {
            n336 = call "GetModuleIndex.vi"("ModuleType"="Scope") -> ("ModuleIndex"=w1028:i32, "Error"=w1026:errorcluster)  [unwired: 9 in]
            n337 = property class="Test.lvclass"(reference=w1024, error in=w1026) -> (reference out=w1016:refnum<class "Test.lvclass">, error out=w1023:errorcluster, "Accessors:ErrorSeverity"=w1019:string, "Accessors:ModuleIDs"=w1027:i32[])
            n338 = Index Array(array=w1027, index=w1028) -> (element=w1022:i32)
            n339 = call "StopAcquisitionRequest.vi"("error in (no error)"=w1023, "ModuleID"=w1022) -> ("error out"=w1018:errorcluster)  [unwired: 9 in]
            n340 = call <userlib>:"AddError.vi"("Severity"=w1019, "Priority"=u8 3, "ErrorArray"=w1017, "error in (no error)"=w1018) -> ("ErrorArray"=w1021:errorcluster[])  [unwired: 6 in, 1 out]
          }
          frame "ScopeAbort" {
            n341 = call "GetModuleIndex.vi"("ModuleType"="Scope") -> ("ModuleIndex"=w1039:i32, "Error"=w1041:errorcluster)  [unwired: 9 in]
            n342 = property class="Test.lvclass"(reference=w1038, error in=w1041) -> (reference out=w1037:refnum<class "Test.lvclass">, error out=w1030:errorcluster, "Accessors:ErrorSeverity"=w1033:string, "Accessors:ModuleIDs"=w1040:i32[])
            n343 = Index Array(array=w1040, index=w1039) -> (element=w1031:i32)
            n344 = call "AbortRequest.vi"("error in (no error)"=w1030, "ModuleID"=w1031) -> ("error out"=w1029:errorcluster)  [unwired: 9 in]
            n345 = call <userlib>:"AddError.vi"("Severity"=w1033, "Priority"=u8 3, "ErrorArray"=w1032, "error in (no error)"=w1029) -> ("ErrorArray"=w1036:errorcluster[])  [unwired: 6 in, 1 out]
          }
          frame "ScopeClose" {
            n346 = call "GetModuleIndex.vi"("ModuleType"="Scope") -> ("ModuleIndex"=w1052:i32, "Error"=w1054:errorcluster)  [unwired: 9 in]
            n347 = property class="Test.lvclass"(reference=w1051, error in=w1054) -> (reference out=w1050:refnum<class "Test.lvclass">, error out=w1043:errorcluster, "Accessors:ErrorSeverity"=w1046:string, "Accessors:ModuleIDs"=w1053:i32[])
            n348 = Index Array(array=w1053, index=w1052) -> (element=w1044:i32)
            n349 = call "CloseRequest.vi"("error in (no error)"=w1043, "ModuleID"=w1044) -> ("error out"=w1042:errorcluster)  [unwired: 9 in]
            n350 = call <userlib>:"AddError.vi"("Severity"=w1046, "Priority"=u8 3, "ErrorArray"=w1045, "error in (no error)"=w1042) -> ("ErrorArray"=w1049:errorcluster[])  [unwired: 6 in, 1 out]
          }
          frame "DigitizerInitialize" {
            n351 = call "GetModuleIndex.vi"("ModuleType"="Digitizer") -> ("ModuleIndex"=w1063:i32, "Error"=w1065:errorcluster)  [unwired: 9 in]
            n352 = property class="Test.lvclass"(reference=w1067, error in=w1065) -> (reference out=w1060:refnum<class "Test.lvclass">, error out=w1061:errorcluster, "Accessors:ErrorSeverity"=w1056:string, "Accessors:ModuleIDs"=w1064:i32[])
            n353 = Index Array(array=w1064, index=w1063) -> (element=w1062:i32)
            n354 = call "InitializeRequest.vi"("error in (no error)"=w1061, "ModuleID"=w1062) -> ("error out"=w1057:errorcluster)  [unwired: 9 in]
            n355 = call <userlib>:"AddError.vi"("Severity"=w1056, "Priority"=u8 3, "ErrorArray"=w1058, "error in (no error)"=w1057) -> ("ErrorArray"=w1059:errorcluster[])  [unwired: 6 in, 1 out]
          }
          frame "DigitizerConfigAcquisition" {
            n356 = call "GetModuleIndex.vi"("ModuleType"="Digitizer") -> ("ModuleIndex"=w1077:i32, "Error"=w1079:errorcluster)  [unwired: 9 in]
            n357 = property class="Test.lvclass"(reference=w1076, error in=w1079) -> (reference out=w1074:refnum<class "Test.lvclass">, error out=w1071:errorcluster, "Accessors:ErrorSeverity"=w1069:string, "Accessors:ModuleIDs"=w1078:i32[])
            n358 = Index Array(array=w1078, index=w1077) -> (element=w1075:i32)
            n359 = call "ConfigAcqRequest.vi"("error in (no error)"=w1071, "ModuleID"=w1075) -> ("error out"=w1072:errorcluster)  [unwired: 9 in]
            n360 = call <userlib>:"AddError.vi"("Severity"=w1069, "Priority"=u8 3, "ErrorArray"=w1070, "error in (no error)"=w1072) -> ("ErrorArray"=w1073:errorcluster[])  [unwired: 6 in, 1 out]
          }
          frame "DigitizerConfigChannels" {
            n361 = call "GetModuleIndex.vi"("ModuleType"="Digitizer") -> ("ModuleIndex"=w1090:i32, "Error"=w1092:errorcluster)  [unwired: 9 in]
            n362 = property class="Test.lvclass"(reference=w1089, error in=w1092) -> (reference out=w1087:refnum<class "Test.lvclass">, error out=w1084:errorcluster, "Accessors:ErrorSeverity"=w1082:string, "Accessors:ModuleIDs"=w1091:i32[])
            n363 = Index Array(array=w1091, index=w1090) -> (element=w1088:i32)
            n364 = call "ConfigChannelsRequest.vi"("error in (no error)"=w1084, "ModuleID"=w1088) -> ("error out"=w1085:errorcluster)  [unwired: 9 in]
            n365 = call <userlib>:"AddError.vi"("Severity"=w1082, "Priority"=u8 3, "ErrorArray"=w1083, "error in (no error)"=w1085) -> ("ErrorArray"=w1086:errorcluster[])  [unwired: 6 in, 1 out]
          }
          frame "DigitizerConfigTrigger" {
            n366 = call "GetModuleIndex.vi"("ModuleType"="Digitizer") -> ("ModuleIndex"=w1103:i32, "Error"=w1105:errorcluster)  [unwired: 9 in]
            n367 = property class="Test.lvclass"(reference=w1102, error in=w1105) -> (reference out=w1100:refnum<class "Test.lvclass">, error out=w1097:errorcluster, "Accessors:ErrorSeverity"=w1095:string, "Accessors:ModuleIDs"=w1104:i32[])
            n368 = Index Array(array=w1104, index=w1103) -> (element=w1101:i32)
            n369 = call "ConfigTrigRequest.vi"("error in (no error)"=w1097, "ModuleID"=w1101) -> ("error out"=w1098:errorcluster)  [unwired: 9 in]
            n370 = call <userlib>:"AddError.vi"("Severity"=w1095, "Priority"=u8 3, "ErrorArray"=w1096, "error in (no error)"=w1098) -> ("ErrorArray"=w1099:errorcluster[])  [unwired: 6 in, 1 out]
          }
          frame "DigitizerWriteSyncInfo" {
            n371 = call "GetModuleIndex.vi"("ModuleType"="Digitizer") -> ("ModuleIndex"=w1117:i32, "Error"=w1119:errorcluster)  [unwired: 9 in]
            n372 = property class="Test.lvclass"(reference=w1116, error in=w1119) -> (reference out=w1114:refnum<class "Test.lvclass">, error out=w1111:errorcluster, "Accessors:ErrorSeverity"=w1109:string, "Accessors:ModuleIDs"=w1118:i32[])
            n373 = Index Array(array=w1118, index=w1117) -> (element=w1115:i32)
            n374 = call "WriteSyncInfoRequest.vi"("error in (no error)"=w1111, "SyncInfo"=w1107, "ModuleID"=w1115) -> ("error out"=w1112:errorcluster)  [unwired: 8 in]
            n375 = call <userlib>:"AddError.vi"("Severity"=w1109, "Priority"=u8 3, "ErrorArray"=w1110, "error in (no error)"=w1112) -> ("ErrorArray"=w1113:errorcluster[])  [unwired: 6 in, 1 out]
          }
          frame "DigitizerFetchWaveforms" {
            n376 = call "GetModuleIndex.vi"("ModuleType"="Digitizer") -> ("ModuleIndex"=w1130:i32, "Error"=w1132:errorcluster)  [unwired: 9 in]
            n377 = property class="Test.lvclass"(reference=w1129, error in=w1132) -> (reference out=w1127:refnum<class "Test.lvclass">, error out=w1124:errorcluster, "Accessors:ErrorSeverity"=w1122:string, "Accessors:ModuleIDs"=w1131:i32[])
            n378 = Index Array(array=w1131, index=w1130) -> (element=w1128:i32)
            n379 = call "FetchWfrmRequest.vi"("error in (no error)"=w1124, "ModuleID"=w1128) -> ("error out"=w1125:errorcluster)  [unwired: 9 in]
            n380 = call <userlib>:"AddError.vi"("Severity"=w1122, "Priority"=u8 3, "ErrorArray"=w1123, "error in (no error)"=w1125) -> ("ErrorArray"=w1126:errorcluster[])  [unwired: 6 in, 1 out]
          }
          frame "DigitizerReadWaveforms" {
            w1140 = "Digitizer" ("ModuleType")
            n381 = call "GetModuleIndex.vi"("ModuleType"=w1140) -> ("ModuleIndex"=w1148:i32, "Error"=w1150:errorcluster)  [unwired: 9 in]
            n382 = property class="Test.lvclass"(reference=w1147, error in=w1150) -> (reference out=w1146:refnum<class "Test.lvclass">, error out=w1135:errorcluster, "Accessors:ErrorSeverity"=w1138:string, "Accessors:ModuleIDs"=w1149:i32[])
            n383 = Index Array(array=w1149, index=w1148) -> (element=w1141:i32)
            n384 = call "GetDigitizerBdcstEvents.vi"("error in (no error)"=w1135) -> ("Event Registration Refnum"=w1136:T7, "error out"=w1134:errorcluster)  [unwired: 9 in]
            n385 = call "ReadWfrmRequest.vi"("error in (no error)"=w1134, "ModuleID"=w1141) -> ("error out"=w1143:errorcluster)  [unwired: 9 in]
            n386 = case shown="Error" w1143 {
              selector: w1143 -> [_ w1165]
              tunnel: w1141 -> [w1161 _]
              tunnel: w1140 -> [w1160 _]
              tunnel: [w1156 w1169] -> w1139
              tunnel: w1142 -> [w1155 w1166]
              tunnel: w1138 -> [_ w1168]
              tunnel: w1137 -> [w1153 _]
              tunnel: w1136 -> [w1151 w1163]
              frame No Error {
                n387 = To Variant(anything=w1151) -> (Variant=w1152:variant)
                n388 = Bundle By Name(cluster=T1 {"ModuleID"=-1, "ModuleType"="", "UserEvtRef"=variant, "ScriptCmd"="", "Timeout"=5000} ("BdcstInfo"), "Timeout"=5000, "ModuleID"=w1161, "ModuleType"=w1160, "ScriptCmd"=w1153, "UserEvtRef"=w1152) -> (w1158:T1)
                n389 = call "Enqueue.vi"("Priority? (f)"=TRUE, "ErrorArray"=w1155, "Data"=w1158, "Message"="GetBdcst") -> ("ErrorArray"=w1156:errorcluster[])  [unwired: 7 in]
              }
              frame Error {
                n390 = Unregister For Events(event registration refnum=w1163, error in=w1165) -> (error out=w1164:errorcluster)
                n391 = call <userlib>:"AddError.vi"("Severity"=w1168, "Priority"=u8 3, "ErrorArray"=w1166, "error in (no error)"=w1164) -> ("ErrorArray"=w1169:errorcluster[])  [unwired: 6 in, 1 out]
              }
            }
            n392 = call <userlib>:"AddError.vi"("Severity"=w1138, "Priority"=u8 3, "ErrorArray"=w1139) -> ("ErrorArray"=w1145:errorcluster[])  [unwired: 7 in, 1 out]
          }
          frame "DigitizerAbort" {
            n393 = call "GetModuleIndex.vi"("ModuleType"="Digitizer") -> ("ModuleIndex"=w1180:i32, "Error"=w1182:errorcluster)  [unwired: 9 in]
            n394 = property class="Test.lvclass"(reference=w1179, error in=w1182) -> (reference out=w1178:refnum<class "Test.lvclass">, error out=w1176:errorcluster, "Accessors:ErrorSeverity"=w1172:string, "Accessors:ModuleIDs"=w1181:i32[])
            n395 = Index Array(array=w1181, index=w1180) -> (element=w1174:i32)
            n396 = call "AbortRequest.vi"("error in (no error)"=w1176, "ModuleID"=w1174) -> ("error out"=w1170:errorcluster)  [unwired: 9 in]
            n397 = call <userlib>:"AddError.vi"("Severity"=w1172, "Priority"=u8 3, "ErrorArray"=w1171, "error in (no error)"=w1170) -> ("ErrorArray"=w1177:errorcluster[])  [unwired: 6 in, 1 out]
          }
          frame "DigitizerClose" {
            n398 = call "GetModuleIndex.vi"("ModuleType"="Digitizer") -> ("ModuleIndex"=w1193:i32, "Error"=w1195:errorcluster)  [unwired: 9 in]
            n399 = property class="Test.lvclass"(reference=w1192, error in=w1195) -> (reference out=w1191:refnum<class "Test.lvclass">, error out=w1189:errorcluster, "Accessors:ErrorSeverity"=w1185:string, "Accessors:ModuleIDs"=w1194:i32[])
            n400 = Index Array(array=w1194, index=w1193) -> (element=w1187:i32)
            n401 = call "CloseRequest.vi"("error in (no error)"=w1189, "ModuleID"=w1187) -> ("error out"=w1183:errorcluster)  [unwired: 9 in]
            n402 = call <userlib>:"AddError.vi"("Severity"=w1185, "Priority"=u8 3, "ErrorArray"=w1184, "error in (no error)"=w1183) -> ("ErrorArray"=w1190:errorcluster[])  [unwired: 6 in, 1 out]
          }
          frame "SensorCreateSession" {
            n403 = call "ExtractModuleID.vi"("ModuleType"="Sensor", "Variant Input"=w1196, "Test.lvclass In"=w1202) -> ("Error Out"=w1201:errorcluster, "ModuleIDs"=w1200:i32, "String"=w1198:string, "Test.lvclass Out"=w1199:refnum<class "Test.lvclass">, "Variant Output"=w1197:variant)  [unwired: 4 in]
            n404 = call "CreateSessionRequest.vi"("error in (no error)"=w1201, "ModuleID"=w1200) -> ("error out"=w1204:errorcluster)  [unwired: 9 in]
            n405 = call <userlib>:"AddError.vi"("Severity"=w1198, "Priority"=u8 3, "ErrorArray"=w1205, "error in (no error)"=w1204) -> ("ErrorArray"=w1207:errorcluster[])  [unwired: 6 in, 1 out]
          }
          frame "SensorConfigure" {
            n406 = call "ExtractModuleID.vi"("ModuleType"="Sensor", "Variant Input"=w1208, "Test.lvclass In"=w1215) -> ("Error Out"=w1210:errorcluster, "ModuleIDs"=w1211:i32, "String"=w1213:string, "Test.lvclass Out"=w1214:refnum<class "Test.lvclass">, "Variant Output"=w1212:variant)  [unwired: 4 in]
            n407 = call "ConfigureRequest.vi"("error in (no error)"=w1210, "ModuleID"=w1211) -> ("error out"=w1209:errorcluster)  [unwired: 9 in]
            n408 = call <userlib>:"AddError.vi"("Severity"=w1213, "Priority"=u8 3, "ErrorArray"=w1217, "error in (no error)"=w1209) -> ("ErrorArray"=w1219:errorcluster[])  [unwired: 6 in, 1 out]
          }
          frame "SensorCloseSession" {
            n409 = call "ExtractModuleID.vi"("ModuleType"="Sensor", "Variant Input"=w1220, "Test.lvclass In"=w1227) -> ("Error Out"=w1223:errorcluster, "ModuleIDs"=w1222:i32, "String"=w1225:string, "Test.lvclass Out"=w1226:refnum<class "Test.lvclass">, "Variant Output"=w1224:variant)  [unwired: 4 in]
            n410 = call "CloseSessionRequest.vi"("error in (no error)"=w1223, "ModuleID"=w1222) -> ("error out"=w1221:errorcluster)  [unwired: 9 in]
            n411 = call <userlib>:"AddError.vi"("Severity"=w1225, "Priority"=u8 3, "ErrorArray"=w1229, "error in (no error)"=w1221) -> ("ErrorArray"=w1231:errorcluster[])  [unwired: 6 in, 1 out]
          }
          frame "SensorStart" {
            n412 = disable-structure shown="Enabled" {
              disable-tunnel: w1242 -> [w1248 w1259]
              disable-tunnel: [w1247 w1258] -> w1241
              disable-tunnel: [w1246 w1256] -> w1239
              disable-tunnel: [w1245 w1252] -> w1237
              disable-tunnel: [w1243 w1257] -> w1236
              disable-tunnel: [_ w1255] -> w1233
              disable-tunnel: w1232 -> [_ w1253]
              frame Disabled {
                n413 = call "GetModuleIndex.vi"("ModuleType"="Sensor") -> ("ModuleIndex"=w1249:i32, "Error"=w1251:errorcluster)  [unwired: 9 in]
                n414 = property class="Test.lvclass"(reference=w1248, error in=w1251) -> (reference out=w1247:refnum<class "Test.lvclass">, error out=w1246:errorcluster, "Accessors:ErrorSeverity"=w1243:string, "Accessors:ModuleIDs"=w1250:i32[])
                n415 = Index Array(array=w1250, index=w1249) -> (element=w1245:i32)
              }
              frame Enabled {
                n416 = call "ExtractModuleID.vi"("ModuleType"="Sensor", "Variant Input"=w1253, "Test.lvclass In"=w1259) -> ("Error Out"=w1256:errorcluster, "ModuleIDs"=w1252:i32, "String"=w1257:string, "Test.lvclass Out"=w1258:refnum<class "Test.lvclass">, "Variant Output"=w1255:variant)  [unwired: 4 in]
              }
            }
            n417 = call "StartDataRequest.vi"("error in (no error)"=w1239, "ModuleID"=w1237) -> ("error out"=w1234:errorcluster)  [unwired: 9 in]
            n418 = call <userlib>:"AddError.vi"("Severity"=w1236, "Priority"=u8 3, "ErrorArray"=w1235, "error in (no error)"=w1234) -> ("ErrorArray"=w1240:errorcluster[])  [unwired: 6 in, 1 out]
          }
          frame "SensorStop" {
            n419 = disable-structure shown="Enabled" {
              disable-tunnel: w1269 -> [w1275 w1285]
              disable-tunnel: [w1274 w1284] -> w1268
              disable-tunnel: [w1273 w1282] -> w1266
              disable-tunnel: [w1272 w1280] -> w1264
              disable-tunnel: [w1270 w1281] -> w1263
              disable-tunnel: w1260 -> [_ w1279]
              frame Disabled {
                n420 = call "GetModuleIndex.vi"("ModuleType"="Sensor") -> ("ModuleIndex"=w1276:i32, "Error"=w1278:errorcluster)  [unwired: 9 in]
                n421 = property class="Test.lvclass"(reference=w1275, error in=w1278) -> (reference out=w1274:refnum<class "Test.lvclass">, error out=w1273:errorcluster, "Accessors:ErrorSeverity"=w1270:string, "Accessors:ModuleIDs"=w1277:i32[])
                n422 = Index Array(array=w1277, index=w1276) -> (element=w1272:i32)
              }
              frame Enabled {
                n423 = call "ExtractModuleID.vi"("ModuleType"="Sensor", "Variant Input"=w1279, "Test.lvclass In"=w1285) -> ("Error Out"=w1282:errorcluster, "ModuleIDs"=w1280:i32, "String"=w1281:string, "Test.lvclass Out"=w1284:refnum<class "Test.lvclass">)  [unwired: 4 in, 1 out]
              }
            }
            n424 = call "StopDataRequest.vi"("error in (no error)"=w1266, "ModuleID"=w1264) -> ("error out"=w1261:errorcluster)  [unwired: 9 in]
            n425 = call <userlib>:"AddError.vi"("Severity"=w1263, "Priority"=u8 3, "ErrorArray"=w1262, "error in (no error)"=w1261) -> ("ErrorArray"=w1267:errorcluster[])  [unwired: 6 in, 1 out]
          }
          frame "AnalysisInitialize" {
            n426 = call "GetModuleIndex.vi"("ModuleType"="Analysis") -> ("ModuleIndex"=w1291:i32, "Error"=w1287:errorcluster)  [unwired: 9 in]
            n427 = property class="Test.lvclass"(reference=w1298, error in=w1287) -> (reference out=w1294:refnum<class "Test.lvclass">, error out=w1286:errorcluster, "Accessors:ErrorSeverity"=w1289:string, "Accessors:ModuleIDs"=w1292:i32[])
            n428 = Index Array(array=w1292, index=w1291) -> (element=w1290:i32)
            n429 = call "InitializeRequest.vi"("error in (no error)"=w1286, "ModuleID"=w1290) -> ("error out"=w1295:errorcluster)  [unwired: 9 in]
            n430 = call <userlib>:"AddError.vi"("Severity"=w1289, "Priority"=u8 3, "ErrorArray"=w1297, "error in (no error)"=w1295) -> ("ErrorArray"=w1296:errorcluster[])  [unwired: 6 in, 1 out]
          }
          frame "AnalysisWriteResultPath" {
            n431 = Variant To Data(type=string[] [], Variant=w1306) -> (data=w1305:string[], error out=w1300:errorcluster)  [unwired: 1 in]
            n432 = Index Array(array=w1305) -> (element=w1304:string)  [unwired: 1 in]
            n433 = String To Path(string=w1304) -> (path=w1303:path)
            n434 = call "GetModuleIndex.vi"("ModuleType"="Analysis") -> ("ModuleIndex"=w1315:i32, "Error"=w1301:errorcluster)  [unwired: 9 in]
            n435 = Merge Errors(w1300, w1301) -> (w1302:errorcluster)
            n436 = property class="Test.lvclass" props=["Accessors:ErrorSeverity", "Accessors:ModuleIDs"](reference=w1314, error in=w1302) -> (reference out=w1313:refnum<class "Test.lvclass">, error out=w1299:errorcluster, "Accessors:ModuleIDs"=w1316:i32[])  [unwired: 1 out]
            n437 = Index Array(array=w1316, index=w1315) -> (element=w1309:i32)
            n438 = call "WriteResultPathRequest.vi"("error in (no error)"=w1299, "ResultPath"=w1303, "ModuleID"=w1309) -> ("error out"=w1310:errorcluster)  [unwired: 8 in]
            n439 = call <userlib>:"AddError.vi"("Priority"=u8 3, "ErrorArray"=w1311, "error in (no error)"=w1310) -> ("ErrorArray"=w1308:errorcluster[])  [unwired: 7 in, 1 out]
          }
          frame "AnalysisWriteWaveforms" {
            n440 = call "GetModuleIndex.vi"("ModuleType"="Analysis") -> ("ModuleIndex"=w1324:i32, "Error"=w1319:errorcluster)  [unwired: 9 in]
            n441 = property class="Test.lvclass"(reference=w1331, error in=w1319) -> (reference out=w1327:refnum<class "Test.lvclass">, error out=w1318:errorcluster, "Accessors:ErrorSeverity"=w1322:string, "Accessors:ModuleIDs"=w1325:i32[])
            n442 = Index Array(array=w1325, index=w1324) -> (element=w1323:i32)
            n443 = call "WriteSampleData.vi"("error in (no error)"=w1318, "SampleDataInput"=w1320, "ModuleID"=w1323) -> ("error out"=w1328:errorcluster)  [unwired: 8 in]
            n444 = call <userlib>:"AddError.vi"("Severity"=w1322, "Priority"=u8 3, "ErrorArray"=w1330, "error in (no error)"=w1328) -> ("ErrorArray"=w1329:errorcluster[])  [unwired: 6 in, 1 out]
          }
          frame "AnalysisWriteSensorData" {
            n445 = call "GetModuleIndex.vi"("ModuleType"="Analysis") -> ("ModuleIndex"=w1338:i32, "Error"=w1333:errorcluster)  [unwired: 9 in]
            n446 = property class="Test.lvclass"(reference=w1345, error in=w1333) -> (reference out=w1341:refnum<class "Test.lvclass">, error out=w1332:errorcluster, "Accessors:ErrorSeverity"=w1336:string, "Accessors:ModuleIDs"=w1339:i32[])
            n447 = Index Array(array=w1339, index=w1338) -> (element=w1337:i32)
            n448 = call "WriteSensorData.vi"("error in (no error)"=w1332, "SensorDataInput"=w1334, "ModuleID"=w1337) -> ("error out"=w1342:errorcluster)  [unwired: 8 in]
            n449 = call <userlib>:"AddError.vi"("Severity"=w1336, "Priority"=u8 3, "ErrorArray"=w1344, "error in (no error)"=w1342) -> ("ErrorArray"=w1343:errorcluster[])  [unwired: 6 in, 1 out]
          }
          frame "AnalysisGetFunctionClass" {
            w1351 = "Analysis"
            n450 = call "GetModuleIndex.vi"("ModuleType"=w1351) -> ("ModuleIndex"=w1358:i32, "Error"=w1356:errorcluster)  [unwired: 9 in]
            n451 = property class="Test.lvclass"(reference=w1360, error in=w1356) -> (reference out=w1357:refnum<class "Test.lvclass">, error out=w1347:errorcluster, "Accessors:ErrorSeverity"=w1353:string, "Accessors:ModuleIDs"=w1359:i32[])
            n452 = Index Array(array=w1359, index=w1358) -> (element=w1352:i32)
            n453 = call "GetFGenBdcstEvents.vi"("error in (no error)"=w1347) -> ("Event Registration Refnum"=w1348:T5, "error out"=w1346:errorcluster)  [unwired: 9 in]
            n454 = call "GetFunctionClassRequest.vi"("error in (no error)"=w1346, "ModuleID"=w1352) -> ("error out"=w1354:errorcluster)  [unwired: 9 in]
            n455 = case shown="No Error" w1354 {
              selector: w1354 -> [_ w1375]
              tunnel: w1352 -> [w1371 _]
              tunnel: w1351 -> [w1370 _]
              tunnel: w1350 -> [w1368 _]
              tunnel: [w1364 w1379] -> w1349
              tunnel: w1355 -> [w1363 w1376]
              tunnel: w1353 -> [_ w1378]
              tunnel: w1348 -> [w1361 w1373]
              frame No Error {
                n456 = To Variant(anything=w1361) -> (Variant=w1369:variant)
                n457 = Bundle By Name(cluster=T1 {"ModuleID"=-1, "ModuleType"="", "UserEvtRef"=variant, "ScriptCmd"="", "Timeout"=5000} ("BdcstInfo"), "Timeout"=5000, "ModuleID"=w1371, "ModuleType"=w1370, "UserEvtRef"=w1369, "ScriptCmd"=w1368) -> (w1366:T1)
                n458 = call "Enqueue.vi"("Priority? (f)"=TRUE, "ErrorArray"=w1363, "Data"=w1366, "Message"="GetBdcst") -> ("ErrorArray"=w1364:errorcluster[])  [unwired: 7 in]
              }
              frame Error {
                n459 = Unregister For Events(event registration refnum=w1373, error in=w1375) -> (error out=w1374:errorcluster)
                n460 = call <userlib>:"AddError.vi"("Severity"=w1378, "Priority"=u8 3, "ErrorArray"=w1376, "error in (no error)"=w1374) -> ("ErrorArray"=w1379:errorcluster[])  [unwired: 6 in, 1 out]
              }
            }
          }
          frame "AnalysisGetFunctionParams" {
            w1385 = "Analysis"
            n461 = call "GetModuleIndex.vi"("ModuleType"=w1385) -> ("ModuleIndex"=w1392:i32, "Error"=w1390:errorcluster)  [unwired: 9 in]
            n462 = property class="Test.lvclass"(reference=w1394, error in=w1390) -> (reference out=w1391:refnum<class "Test.lvclass">, error out=w1381:errorcluster, "Accessors:ErrorSeverity"=w1387:string, "Accessors:ModuleIDs"=w1393:i32[])
            n463 = Index Array(array=w1393, index=w1392) -> (element=w1386:i32)
            n464 = call "GetFGenBdcstEvents.vi"("error in (no error)"=w1381) -> ("Event Registration Refnum"=w1382:T5, "error out"=w1380:errorcluster)  [unwired: 9 in]
            n465 = call "GetFunctionParamsRequest.vi"("error in (no error)"=w1380, "ModuleID"=w1386) -> ("error out"=w1388:errorcluster)  [unwired: 9 in]
            n466 = case shown="Error" w1388 {
              selector: w1388 -> [_ w1409]
              tunnel: w1386 -> [w1405 _]
              tunnel: w1385 -> [w1404 _]
              tunnel: w1384 -> [w1402 _]
              tunnel: [w1398 w1413] -> w1383
              tunnel: w1389 -> [w1397 w1410]
              tunnel: w1387 -> [_ w1412]
              tunnel: w1382 -> [w1395 w1407]
              frame No Error {
                n467 = To Variant(anything=w1395) -> (Variant=w1403:variant)
                n468 = Bundle By Name(cluster=T1 {"ModuleID"=-1, "ModuleType"="", "UserEvtRef"=variant, "ScriptCmd"="", "Timeout"=5000} ("BdcstInfo"), "Timeout"=5000, "ModuleID"=w1405, "ModuleType"=w1404, "UserEvtRef"=w1403, "ScriptCmd"=w1402) -> (w1400:T1)
                n469 = call "Enqueue.vi"("Priority? (f)"=TRUE, "ErrorArray"=w1397, "Data"=w1400, "Message"="GetBdcst") -> ("ErrorArray"=w1398:errorcluster[])  [unwired: 7 in]
              }
              frame Error {
                n470 = Unregister For Events(event registration refnum=w1407, error in=w1409) -> (error out=w1408:errorcluster)
                n471 = call <userlib>:"AddError.vi"("Severity"=w1412, "Priority"=u8 3, "ErrorArray"=w1410, "error in (no error)"=w1408) -> ("ErrorArray"=w1413:errorcluster[])  [unwired: 6 in, 1 out]
              }
            }
          }
          frame "AnalysisGetState" {
            w1419 = "Analysis"
            n472 = call "GetModuleIndex.vi"("ModuleType"=w1419) -> ("ModuleIndex"=w1426:i32, "Error"=w1424:errorcluster)  [unwired: 9 in]
            n473 = property class="Test.lvclass"(reference=w1428, error in=w1424) -> (reference out=w1425:refnum<class "Test.lvclass">, error out=w1415:errorcluster, "Accessors:ErrorSeverity"=w1421:string, "Accessors:ModuleIDs"=w1427:i32[])
            n474 = Index Array(array=w1427, index=w1426) -> (element=w1420:i32)
            n475 = call "GetAnalysisBdcstEvents.vi"("error in (no error)"=w1415) -> ("Event Registration Refnum"=w1416:refnum<event-registration>, "error out"=w1414:errorcluster)  [unwired: 9 in]
            n476 = call "GetStateRequest.vi"("error in (no error)"=w1414, "ModuleID"=w1420) -> ("error out"=w1422:errorcluster)  [unwired: 9 in]
            n477 = case shown="No Error" w1422 {
              selector: w1422 -> [_ w1444]
              tunnel: w1420 -> [w1439 _]
              tunnel: w1419 -> [w1438 _]
              tunnel: w1418 -> [w1436 _]
              tunnel: [w1432 w1445] -> w1417
              tunnel: w1423 -> [w1431 w1441]
              tunnel: w1421 -> [_ w1443]
              tunnel: w1416 -> [w1429 _]
              frame No Error {
                n478 = To Variant(anything=w1429) -> (Variant=w1437:variant)
                n479 = Bundle By Name(cluster=T1 {"ModuleID"=-1, "ModuleType"="", "UserEvtRef"=variant, "ScriptCmd"="", "Timeout"=5000} ("BdcstInfo"), "Timeout"=10000, "ModuleID"=w1439, "ModuleType"=w1438, "UserEvtRef"=w1437, "ScriptCmd"=w1436) -> (w1434:T1)
                n480 = call "Enqueue.vi"("Priority? (f)"=TRUE, "ErrorArray"=w1431, "Data"=w1434, "Message"="GetBdcst") -> ("ErrorArray"=w1432:errorcluster[])  [unwired: 7 in]
              }
              frame Error {
                n481 = call <userlib>:"AddError.vi"("Severity"=w1443, "Priority"=u8 3, "ErrorArray"=w1441, "error in (no error)"=w1444) -> ("ErrorArray"=w1445:errorcluster[])  [unwired: 6 in, 1 out]
              }
            }
          }
          frame "AnalysisSetFunctionClass" {
            n482 = call "GetModuleIndex.vi"("ModuleType"="Analysis") -> ("ModuleIndex"=w1452:i32, "Error"=w1447:errorcluster)  [unwired: 9 in]
            n483 = property class="Test.lvclass"(reference=w1459, error in=w1447) -> (reference out=w1455:refnum<class "Test.lvclass">, error out=w1446:errorcluster, "Accessors:ErrorSeverity"=w1450:string, "Accessors:ModuleIDs"=w1453:i32[])
            n484 = Index Array(array=w1453, index=w1452) -> (element=w1451:i32)
            n485 = call "SetFunctionClassRequest.vi"("error in (no error)"=w1446, "FunctionClass"=w1448, "ModuleID"=w1451) -> ("error out"=w1456:errorcluster)  [unwired: 8 in]
            n486 = call <userlib>:"AddError.vi"("Severity"=w1450, "Priority"=u8 3, "ErrorArray"=w1458, "error in (no error)"=w1456) -> ("ErrorArray"=w1457:errorcluster[])  [unwired: 6 in, 1 out]
          }
          frame "AnalysisSetFunctionParams" {
            n487 = call "GetModuleIndex.vi"("ModuleType"="Analysis") -> ("ModuleIndex"=w1466:i32, "Error"=w1461:errorcluster)  [unwired: 9 in]
            n488 = property class="Test.lvclass"(reference=w1473, error in=w1461) -> (reference out=w1469:refnum<class "Test.lvclass">, error out=w1460:errorcluster, "Accessors:ErrorSeverity"=w1464:string, "Accessors:ModuleIDs"=w1467:i32[])
            n489 = Index Array(array=w1467, index=w1466) -> (element=w1465:i32)
            n490 = call "SetFunctionParamsRequest.vi"("error in (no error)"=w1460, "FunctionParams"=w1462, "ModuleID"=w1465) -> ("error out"=w1470:errorcluster)  [unwired: 8 in]
            n491 = call <userlib>:"AddError.vi"("Severity"=w1464, "Priority"=u8 3, "ErrorArray"=w1472, "error in (no error)"=w1470) -> ("ErrorArray"=w1471:errorcluster[])  [unwired: 6 in, 1 out]
          }
          frame "AnalysisAbort" {
            n492 = call "GetModuleIndex.vi"("ModuleType"="Analysis") -> ("ModuleIndex"=w1479:i32, "Error"=w1475:errorcluster)  [unwired: 9 in]
            n493 = property class="Test.lvclass"(reference=w1486, error in=w1475) -> (reference out=w1482:refnum<class "Test.lvclass">, error out=w1474:errorcluster, "Accessors:ErrorSeverity"=w1477:string, "Accessors:ModuleIDs"=w1480:i32[])
            n494 = Index Array(array=w1480, index=w1479) -> (element=w1478:i32)
            n495 = call "AbortRequest.vi"("error in (no error)"=w1474, "ModuleID"=w1478) -> ("error out"=w1483:errorcluster)  [unwired: 9 in]
            n496 = call <userlib>:"AddError.vi"("Severity"=w1477, "Priority"=u8 3, "ErrorArray"=w1485, "error in (no error)"=w1483) -> ("ErrorArray"=w1484:errorcluster[])  [unwired: 6 in, 1 out]
          }
          frame "AcPwrInit" {
            n497 = call "ExtractModuleID.vi"("ModuleType"="AcPwr", "Variant Input"=w1492, "Test.lvclass In"=w1493) -> ("Error Out"=w1488:errorcluster, "ModuleIDs"=w1489:i32, "String"=w1490:string, "Test.lvclass Out"=w1491:refnum<class "Test.lvclass">)  [unwired: 4 in, 1 out]
            n498 = call "InitializeRequest.vi"("error in (no error)"=w1488, "ModuleID"=w1489) -> ("error out"=w1495:errorcluster)  [unwired: 9 in]
            n499 = call <userlib>:"AddError.vi"("Severity"=w1490, "Priority"=u8 3, "ErrorArray"=w1497, "error in (no error)"=w1495) -> ("ErrorArray"=w1496:errorcluster[])  [unwired: 6 in, 1 out]
          }
          frame "AcPwrGet" {
            n500 = call "ExtractModuleID.vi"("ModuleType"="AcPwr", "Variant Input"=w1519, "Test.lvclass In"=w1520) -> ("Error Out"=w1517:errorcluster, "ModuleIDs"=w1501:i32, "String"=w1503:string, "Test.lvclass Out"=w1505:refnum<class "Test.lvclass">, "Variant Output"=w1518:variant)  [unwired: 4 in]
            n501 = Variant To Data(error in=w1517, type=string[] [], Variant=w1518) -> (data=w1514:string[], error out=w1516:errorcluster)
            n502 = Index Array(array=w1514) -> (element #2=w1513:string)  [unwired: 2 in, 1 out]
            n503 = To Variant(anything=w1513) -> (Variant=w1512:variant)
            n504 = call "GetSettingsRequest.vi"("Error In"=w1516, "SettingsToGet"=w1512, "ModuleID"=w1501) -> ("Error Out"=w1511:errorcluster)  [unwired: 8 in]
            n505 = call "GetAcPwrBdcstEvents.vi"("error in (no error)"=w1511) -> ("Event Registration Refnum"=w1506:T8, "error out"=w1507:errorcluster)  [unwired: 9 in]
            n506 = case shown="No Error" w1507 {
              selector: w1507 -> [w1526 w1543]
              tunnel: w1501 -> [w1536 _]
              tunnel: "AcPwr" ("ModuleType") -> [w1535 _]
              tunnel: w1499 -> [w1534 _]
              tunnel: w1510 -> [w1530 w1541]
              tunnel: w1506 -> [w1528 w1542]
              tunnel: [w1527 w1541] -> w1509
              tunnel: [w1526 w1540] -> w1508
              tunnel: w1505 -> [w1525 w1539]
              tunnel: [w1525 w1539] -> w1504
              tunnel: w1503 -> [w1524 w1538]
              tunnel: [w1524 w1538] -> w1502
              frame No Error {
                n507 = To Variant(anything=w1528) -> (Variant=w1523:variant)
                n508 = Bundle By Name(cluster=T1 {"ModuleID"=-1, "ModuleType"="", "UserEvtRef"=variant, "ScriptCmd"="", "Timeout"=5000} ("BdcstInfo"), "Timeout"=5000, "ModuleID"=w1536, "ModuleType"=w1535, "ScriptCmd"=w1534, "UserEvtRef"=w1523) -> (w1532:T1)
                n509 = call "Enqueue.vi"("Priority? (f)"=TRUE, "ErrorArray"=w1530, "Data"=w1532, "Message"="GetBdcst") -> ("ErrorArray"=w1527:errorcluster[])  [unwired: 7 in]
              }
              frame Error {
                n510 = Unregister For Events(event registration refnum=w1542, error in=w1543) -> (error out=w1540:errorcluster)
              }
            }
            n511 = call <userlib>:"AddError.vi"("Severity"=w1502, "Priority"=u8 3, "ErrorArray"=w1509, "error in (no error)"=w1508) -> ("ErrorArray"=w1522:errorcluster[])  [unwired: 6 in, 1 out]
          }
          frame "AcPwrSet" {
            n512 = call "ExtractModuleID.vi"("ModuleType"="AcPwr", "Variant Input"=w1558, "Test.lvclass In"=w1559) -> ("Error Out"=w1553:errorcluster, "ModuleIDs"=w1555:i32, "String"=w1556:string, "Test.lvclass Out"=w1557:refnum<class "Test.lvclass">, "Variant Output"=w1554:variant)  [unwired: 4 in]
            n513 = Variant To Data(error in=w1553, type=string[] [], Variant=w1554) -> (data=w1550:string[], error out=w1552:errorcluster)
            n514 = Index Array(array=w1550) -> (element #2=w1548:string, element #3=w1547:string)  [unwired: 3 in, 1 out]
            n515 = Build Array(w1548, w1547) -> (w1546:string[])
            n516 = To Variant(anything=w1546) -> (Variant=w1549:variant)
            n517 = call "SetSettingsRequest.vi"("Error In"=w1552, "Data"=w1549, "ModuleID"=w1555) -> ("Error Out"=w1561:errorcluster)  [unwired: 8 in]
            n518 = call <userlib>:"AddError.vi"("Severity"=w1556, "Priority"=u8 3, "ErrorArray"=w1563, "error in (no error)"=w1561) -> ("ErrorArray"=w1562:errorcluster[])  [unwired: 6 in, 1 out]
          }
          frame "AcPwrConfig" {
            n519 = call "ExtractModuleID.vi"("ModuleType"="AcPwr", "Variant Input"=w1569, "Test.lvclass In"=w1570) -> ("Error Out"=w1566:errorcluster, "ModuleIDs"=w1565:i32, "String"=w1567:string, "Test.lvclass Out"=w1568:refnum<class "Test.lvclass">)  [unwired: 4 in, 1 out]
            n520 = call "ConfigDeviceRequest.vi"("Error In"=w1566, "ModuleID"=w1565) -> ("Error Out"=w1572:errorcluster)  [unwired: 9 in]
            n521 = call <userlib>:"AddError.vi"("Severity"=w1567, "Priority"=u8 3, "ErrorArray"=w1574, "error in (no error)"=w1572) -> ("ErrorArray"=w1573:errorcluster[])  [unwired: 6 in, 1 out]
          }
          frame "AcPwrDeviceOn" {
            n522 = call "ExtractModuleID.vi"("ModuleType"="AcPwr", "Variant Input"=w1576, "Test.lvclass In"=w1581) -> ("Error Out"=w1577:errorcluster, "ModuleIDs"=w1578:i32, "String"=w1579:string, "Test.lvclass Out"=w1580:refnum<class "Test.lvclass">)  [unwired: 4 in, 1 out]
            n523 = call "DeviceOnRequest.vi"("Error In"=w1577, "ModuleID"=w1578) -> ("Error Out"=w1583:errorcluster)  [unwired: 9 in]
            n524 = call <userlib>:"AddError.vi"("Severity"=w1579, "Priority"=u8 3, "ErrorArray"=w1585, "error in (no error)"=w1583) -> ("ErrorArray"=w1584:errorcluster[])  [unwired: 6 in, 1 out]
          }
          frame "AcPwrDeviceOff" {
            n525 = call "ExtractModuleID.vi"("ModuleType"="AcPwr", "Variant Input"=w1587, "Test.lvclass In"=w1592) -> ("Error Out"=w1588:errorcluster, "ModuleIDs"=w1589:i32, "String"=w1590:string, "Test.lvclass Out"=w1591:refnum<class "Test.lvclass">)  [unwired: 4 in, 1 out]
            n526 = call "DeviceOffRequest.vi"("Error In"=w1588, "ModuleID"=w1589) -> ("Error Out"=w1594:errorcluster)  [unwired: 9 in]
            n527 = call <userlib>:"AddError.vi"("Severity"=w1590, "Priority"=u8 3, "ErrorArray"=w1596, "error in (no error)"=w1594) -> ("ErrorArray"=w1595:errorcluster[])  [unwired: 6 in, 1 out]
          }
          frame "AcPwrStartMeas" {
            n528 = call "ExtractModuleID.vi"("ModuleType"="AcPwr", "Variant Input"=w1603, "Test.lvclass In"=w1607) -> ("Error Out"=w1602:errorcluster, "ModuleIDs"=w1604:i32, "String"=w1605:string, "Test.lvclass Out"=w1606:refnum<class "Test.lvclass">, "Variant Output"=w1601:variant)  [unwired: 4 in]
            n529 = Variant To Data(error in=w1602, type=string[] [], Variant=w1601) -> (data=w1610:string[], error out=w1600:errorcluster)
            n530 = Index Array(array=w1610, index=1) -> (element=w1599:string)
            n531 = Decimal String To Number(string=w1599) -> (number=w1608:i32)  [unwired: 2 in, 1 out]
            n532 = call "StartMeasurementRequest.vi"("Error In"=w1600, "Program Number"=w1608, "ModuleID"=w1604) -> ("Error Out"=w1611:errorcluster)  [unwired: 8 in]
            n533 = call <userlib>:"AddError.vi"("Severity"=w1605, "Priority"=u8 3, "ErrorArray"=w1614, "error in (no error)"=w1611) -> ("ErrorArray"=w1613:errorcluster[])  [unwired: 6 in, 1 out]
          }
          frame "AcPwrStopMeas" {
            n534 = call "ExtractModuleID.vi"("ModuleType"="AcPwr", "Variant Input"=w1620, "Test.lvclass In"=w1621) -> ("Error Out"=w1616:errorcluster, "ModuleIDs"=w1617:i32, "String"=w1618:string, "Test.lvclass Out"=w1619:refnum<class "Test.lvclass">)  [unwired: 4 in, 1 out]
            n535 = call "StopMeasurementRequest.vi"("Error In"=w1616, "ModuleID"=w1617) -> ("Error Out"=w1622:errorcluster)  [unwired: 9 in]
            n536 = call <userlib>:"AddError.vi"("Severity"=w1618, "Priority"=u8 3, "ErrorArray"=w1625, "error in (no error)"=w1622) -> ("ErrorArray"=w1624:errorcluster[])  [unwired: 6 in, 1 out]
          }
          frame "AcPwrReset" {
            n537 = call "ExtractModuleID.vi"("ModuleType"="AcPwr", "Variant Input"=w1631, "Test.lvclass In"=w1632) -> ("Error Out"=w1627:errorcluster, "ModuleIDs"=w1628:i32, "String"=w1629:string, "Test.lvclass Out"=w1630:refnum<class "Test.lvclass">)  [unwired: 4 in, 1 out]
            n538 = call "ResetRequest.vi"("Error In"=w1627, "ModuleID"=w1628) -> ("Error Out"=w1633:errorcluster)  [unwired: 9 in]
            n539 = call <userlib>:"AddError.vi"("Severity"=w1629, "Priority"=u8 3, "ErrorArray"=w1636, "error in (no error)"=w1633) -> ("ErrorArray"=w1635:errorcluster[])  [unwired: 6 in, 1 out]
          }
          frame "AcPwrClose" {
            n540 = call "ExtractModuleID.vi"("ModuleType"="AcPwr", "Variant Input"=w1641, "Test.lvclass In"=w1643) -> ("Error Out"=w1640:errorcluster, "ModuleIDs"=w1639:i32, "String"=w1638:string, "Test.lvclass Out"=w1642:refnum<class "Test.lvclass">)  [unwired: 4 in, 1 out]
            n541 = call "CloseRequest.vi"("error in (no error)"=w1640, "ModuleID"=w1639) -> ("error out"=w1644:errorcluster)  [unwired: 9 in]
            n542 = call <userlib>:"AddError.vi"("Severity"=w1638, "Priority"=u8 3, "ErrorArray"=w1647, "error in (no error)"=w1644) -> ("ErrorArray"=w1646:errorcluster[])  [unwired: 6 in, 1 out]
          }
          frame "GetSysTime" {
            n543 = Get Date/Time In Seconds() -> (seconds since 1Jan1904=w1655:timestamp)
            n544 = call "DeQue.vi"("ErrorArray"=w1653) -> ("ErrorArray"=w1652:errorcluster[], "Message"=w1651:string)  [unwired: 8 in, 1 out]
            n545 = To Double Precision Float(number=w1655) -> (double precision float=w1650:dbl)
            n546 = call "Enqueue.vi"("Priority? (f)"=TRUE, "ErrorArray"=w1652, "Data"=w1650, "Message"=w1651) -> ("ErrorArray"=w1649:errorcluster[])  [unwired: 7 in]
          }
          frame "LoopConfigStopCond" {
            n547 = call "LoopConfigStopCond.vi"("Error"=w1660, "StopCondition"=w1659, "Test.lvclass"=w1658) -> ("Error"=w1657:errorcluster[], "Test.lvclass"=w1656:refnum<class "Test.lvclass">)  [unwired: 7 in]
          }
          frame "GetLoopScript" {
            n548 = Variant To Data(type=string[] [], Variant=w1670) -> (data=w1668:string[])  [unwired: 1 in, 1 out]
            n549 = call "GetLoopScript.vi"("Script"="LoopScript", "ErrorArray"=w1671, "ModuleNames"=w1668, "Test.lvclass"=w1667) -> ("ErrorArray"=w1665:errorcluster[], "Test.lvclass"=w1666:refnum<class "Test.lvclass">)  [unwired: 6 in]
            n550 = call "Enqueue.vi"("Priority? (f)"=TRUE, "ErrorArray"=w1665, "Message"="LoopTop") -> ("ErrorArray"=w1664:errorcluster[])  [unwired: 8 in]
          }
          frame "LoopSetStopCondition" {
            n551 = call-dynamic "LoopSetStopCondition.vi"("ErrorArray"=w1676, "StopCondition"=w1675, "Test.lvclass"=w1674) -> ("ErrorArray"=w1672:errorcluster[], "Test.lvclass"=w1673:refnum<class "Test.lvclass">)  [unwired: 7 in]
          }
          frame "LoopTop" {
            n552 = property class="Test.lvclass"(reference=w1682) -> (reference out=w1677:refnum<class "Test.lvclass">, "Accessors:LoopScript"=w1681:string[])  [unwired: 1 in, 1 out]
            n553 = Reverse 1D Array(array=w1681) -> (reversed array=w1678:string[])
            n554 = for {
              shift-right: [w1684] -> w1679
              shift-left: w1680 -> [w1685]
              tunnel: w1678 -> [w1683] mode=indexing
              n555 = Spreadsheet String To Array(delimiter (Tab)=",", format string="%s", spreadsheet string=w1683, array type (2D Dbl)=string[] []) -> (array=w1691:string[])
              n556 = Split 1D Array(array=w1691, index=1) -> (first subarray=w1692:string[], second subarray=w1693:string[])
              n557 = To Variant(anything=w1693) -> (Variant=w1687:variant)
              n558 = Index Array(array=w1692) -> (element=w1686:string)  [unwired: 1 in]
              n559 = call "Enqueue.vi"("Priority? (f)"=TRUE, "ErrorArray"=w1685, "Data"=w1687, "Message"=w1686) -> ("ErrorArray"=w1684:errorcluster[])  [unwired: 7 in]
            }
          }
          frame "LoopUntilDone" {
            # "This is where child classes may add other loop stop conditions"
            n560 = call-dynamic "LoopStopTest.vi"("ErrorArray"=w1702, "LoopStopCondition"=w1701, "Test.lvclass"=w1700) -> ("ErrorArray"=w1697:errorcluster[], "StopLoop?"=w1699:bool, "Test.lvclass"=w1698:refnum<class "Test.lvclass">)  [unwired: 6 in]
            n561 = case shown="False" w1699 {
              tunnel: w1697 -> [w1705 w1707]
              tunnel: [w1706 w1707] -> w1696
              frame False {
                n562 = call "Enqueue.vi"("Priority? (f)"=TRUE, "ErrorArray"=w1705, "Message"="LoopTop") -> ("ErrorArray"=w1706:errorcluster[])  [unwired: 8 in]
              }
              frame True {
              }
            }
          }
          frame Default {
            n563 = property class="Test.lvclass"(reference=w1717) -> (reference out=w1710:refnum<class "Test.lvclass">, error out=w1708:errorcluster, "Accessors:ErrorSeverity"=w1714:string)  [unwired: 1 in]
            n564 = xnode "Error Ring"("parameter 0"=w1711) -> ("error out"=w1712:errorcluster)
            n565 = Merge Errors(w1712, w1708) -> (w1709:errorcluster)
            n566 = call <userlib>:"AddError.vi"("Severity"=w1714, "Priority"=u8 3, "ErrorArray"=w1716, "error in (no error)"=w1709) -> ("ErrorArray"=w1715:errorcluster[])  [unwired: 6 in, 1 out]
          }
        }
        n567 = call "HandleError.vi"("ErrorArray"=w63) -> ("ErrorArray"=w68:errorcluster[], "Stop"=w69:bool)  [unwired: 8 in, 1 out]
        n568 = Or(x=w69, y=w65) -> (x .or. y?=w60:bool)
        n569 = call <extravilib>:"Write.vi"("element"=w60) -> ("channel"=w55:T9)  [unwired: 1 out]
      }
      n570 = while {
        tunnel: w24 -> [_]
        tunnel: w23 -> [w46]
        tunnel: w22 -> [w44]
        tunnel: [w39] -> w21
        tunnel: [w38] -> w19
        tunnel: w11 -> [w36]
        stop <- w35 stop-if-true
        # "Handles all module errors"
        n571 = local read "ErrorSeverity"() -> (w41:string)
        n572 = event shown="[1] Timeout" {
          selector: w46 -> [_ _]
          dyn-events: [_ _] -> w39
          timeout: 50 -> [_ _]
          tunnel: [w51 _] -> w45
          event User Event {
            n573 = event-data() -> ("Data"=w54:variant)  [unwired: 1 in]
            n574 = Variant To Data(type=errorcluster {"status"=FALSE, "code"=0, "source"=""} ("error constant"), Variant=w54) -> (data=w52:errorcluster, error out=w50:errorcluster)  [unwired: 1 in]
            n575 = Merge Errors(w52, w50) -> (w51:errorcluster)
          }
          event Timeout {
            n576 = event-data() -> ()  [unwired: 1 in, 1 out]
          }
        }
        n577 = call <userlib>:"AddError.vi"("Severity"=w41, "Priority"=u8 3, "ErrorArray"=w44, "error in (no error)"=w45) -> ("ErrorArray"=w40:errorcluster[])  [unwired: 6 in, 1 out]
        n578 = call <extravilib>:"Read.vi"("channel"=w36) -> ("element"=w35:bool)  [unwired: 1 in, 1 out]
        n579 = Empty Array?(array=w40) -> (empty?=w37:bool)
        n580 = case shown="True" w37 {
          tunnel: w40 -> [w47 w49]
          tunnel: [w48 w49] -> w38
          frame False {
            n581 = call "HandleError.vi"("ErrorArray"=w47) -> ("ErrorArray"=w48:errorcluster[])  [unwired: 8 in, 2 out]
          }
          frame True {
          }
        }
      }
      n582 = Unregister For Events(event registration refnum=w21) -> (error out=w20:errorcluster)  [unwired: 1 in]
      n583 = call <userlib>:"AddError.vi"("Severity"="Critical", "Priority"=u8 1, "ErrorArray"=w19, "error in (no error)"=w20) -> ("ErrorArray"=w18:errorcluster[])  [unwired: 6 in, 1 out]
      n584 = call "ObtainQueue.vi"("Destroy? (f)"=TRUE, "ErrorArray"=w28) -> ("ErrorArray."=w27:errorcluster[])  [unwired: 8 in, 1 out]
      n585 = Build Array (concatenate)(w18, w27) -> (w12:errorcluster[])
    }
  }
  "Test.lvclass" <- w6
  "Data" <- w4
  "ErrorArray" <- w1
